vi "Plugin_GUI.vi"(8 "error in (no error)":errorcluster, 10 "Communication Interface":refnum<class "Communication Interface.lvclass">, 11 "Process in":refnum<class "Process.lvclass">) -> (0 "error out":errorcluster, 3 "Process out":refnum<class "Process.lvclass">)   [LabVIEW 2020, in "Plugin.lvlib" / "Plugin_UI.lvclass"]
doc: "Configuration User Interface for Plugin"
uses:
  Plugin_UI.lvclass
  builds/Libraries/Shared GUI Library.lvlibp/Shared GUI Library/Instrument Settings/Interface/Serial Interafce.ctl
  builds/Libraries/LabSys Framework.lvlibp/Process/Process/Process.lvclass
  builds/Libraries/LabSys Framework.lvlibp/Process/Communication Interface/Communication Interface.lvclass
  builds/Libraries/design.lvlibp/GUI/Design/CustomButtons/scale_32.ctl
  Output Channel Config.ctl
  builds/Libraries/Shared GUI Library.lvlibp/Shared GUI Library/Instrument Settings/Interface/Settings Container.ctl
  builds/Libraries/Shared GUI Library.lvlibp/Shared GUI Library/Device Meta Data Cluster/DeviceMetaDataCluster.ctl
  builds/Libraries/design.lvlibp/GUI/Design/CustomButtons/LineType/clear_list_l.ctl
  builds/Libraries/design.lvlibp/GUI/Design/CustomButtons/LineType/play_32.ctl
  builds/Libraries/Shared GUI Library.lvlibp/Shared GUI Library/Queue Driver/Typedefs/Operation.ctl
  builds/Libraries/LabSys Framework.lvlibp/Configurable Data Node/Configuration UI Event Interface/Configuration UI Event Interface.lvclass
  Main Cluster.ctl
  C:/SVN_LabSys/labsys_lvcode/LabSys_SourceCode/builds/Libraries/LabSys Framework.lvlibp/Configurable Data Node/Configuration Interface/Configuration Interface.lvclass
  C:/SVN_LabSys/labsys_lvcode/LabSys_SourceCode/builds/Libraries/LabSys Framework.lvlibp/Process/Process/Process.lvclass
  builds/Libraries/Shared GUI Library.lvlibp/Shared GUI Library/Producer error/Error type.ctl
  builds/Libraries/Shared GUI Library.lvlibp/1abvi3w/vi.lib/event_ctls.llb/lveventtype.ctl
  <vilib>/Utility/miscctls.llb/LVPointTypeDef.ctl
  builds/Libraries/LabSys Framework.lvlibp/Error Manager/Error Manager/Error Levels.ctl
  builds/Libraries/Shared GUI Library.lvlibp/Shared GUI Library/Queue Driver/Typedefs/Data.ctl
  Plugin_UI.lvclass/Plugin_UI.ctl
  builds/Libraries/Shared GUI Library.lvlibp/Shared GUI Library/Instrument Settings/Interface/Interface Type.ctl
  <vilib>/Utility/miscctls.llb/LVRowAndColumnTypeDef.ctl
  Write Input Channels[].vi
  Write Output Channels[].vi
  Read Output Channels[].vi
  Read Input Channels[].vi
  Channels/Output Channels/Output Channels.lvclass
  C:/SVN_LabSys/labsys_lvcode/LabSys_SourceCode/Plugin Template/Source/Code/Channels/Plugin_Channels.lvclass
  Channels/Input Channels/Input Channels.lvclass
  builds/Libraries/LabSys Framework.lvlibp/Configurable Data Node/Configuration Interface/Read Module Configuration.vi
  builds/Libraries/LabSys Framework.lvlibp/Configuration Storage/Module Configuration/Read Module Name.vi
  builds/Libraries/LabSys Framework.lvlibp/Configuration Storage/Module Configuration/Get Lookup Tables.vi
  builds/Libraries/LabSys Framework.lvlibp/Configuration Storage/Module Configuration/Get Scaling Functions.vi
  builds/Libraries/LabSys Framework.lvlibp/Configurable Data Node/Configuration Interface/Write Module Configuration.vi
  Write Lookup Tables.vi
  Write Scaling Functions.vi
  Read Lookup Tables.vi
  Read Scaling Functions.vi
  builds/Libraries/LabSys Framework.lvlibp/Configuration Storage/Module Configuration/Set Lookup Tables.vi
  builds/Libraries/LabSys Framework.lvlibp/Configuration Storage/Module Configuration/Set Scaling Functions.vi
  builds/Libraries/LabSys Framework.lvlibp/Process/Process/Read Error Manager.vi
  builds/Libraries/LabSys Framework.lvlibp/Configuration Storage/Module Configuration/Module Configuration.lvclass
  <vilib>/ErrorRing/Error Ring.xnode
  builds/Libraries/LabSys Framework.lvlibp/Error Manager/Error Manager/Error Manager.lvclass
  Controller_Class/Plugin_Controller.lvclass
  builds/Libraries/Shared GUI Library.lvlibp/Shared GUI Library/Queue Driver/Queue Driver.lvlib
  builds/Libraries/Shared GUI Library.lvlibp
  builds/Libraries/LabSys Framework.lvlibp/Configurable Data Node/Configuration Interface/Configuration Interface.lvclass
  C:/SVN_LabSys/labsys_lvcode/LabSys_SourceCode/builds/Libraries/LabSys Framework.lvlibp/Process/Communication Interface/Communication Interface.lvclass
  builds/Libraries/design.lvlibp
panel:
  in  "Label":string="Plugin_UI"
  in  "scale":T1
  in  "setDefault":bool
  in  "Tab Control":enum32{"Interface", "Channels", "Test"}(tab)
  in  "Timeout (ms)":i32=5000
  in  "VISA":refnum<visa-resource-name>
  in  "Device IP":string="192.168.1.1.100"
  in  "Device Meta Data":T2
  in  "Interface Type":T4=enum."Serial"
  in  "Serial Interface":T5={"Baud Rate"=9600, "Data Bits "=8, "Parity"=enum."None", "Stop Bits"=10} {"Stop Bits" items=["1.0", "1.5", "2.0"]; "Baud Rate" items=["1200"=1200, "2400"=2400, "4800"=4800, "9600"=9600, "19200"=19200, "38400"=38400, "57600"=57600, "115200"=115200]}
  in  "Refresh Time (ms)":dbl=1000.0 min=100.0 max=10000.0 step=10.0
  in  "Select All?":enum8{"False", "True", "Mixed"}(c332)
  in  "Measurement Channels":i32(listbox)=5
  in  "Output Settings":T6={"Enable Output"=FALSE, "Channel Name"="", "Value"=1.0, "Unit"=""} {"Value" min=-422.2 max=422.2 step=1.0 format="%#.1f"}
  in  "Start Test":T7 caption="Test"
  out "Test Result":i32(listbox)=-1
  # "#PluginSpecificEdits_UI_1 \nUpdate Plugin name"
  # "Hardware Configuration"
  # "#In Hardware Configuration controls are not locked Because #PluginSpecificEdits__UI_3"
  # "#PluginSpecificEdits_UI_2 \n1. Delete Hardware configuration Which is not required and update according to the \nInterface type"
  # "Device Meta Data"
  # "Input Settings"
  # "#PluginSpecificEdits_UI_16\n Add or Remove Pluginspecific parameters in O/P Settings"
  # "Output Settings"
  # "#PluginSpecificEdits_UI_24 \nHeader section based on available pluginSpecific Settings"
  # "Functional Test"
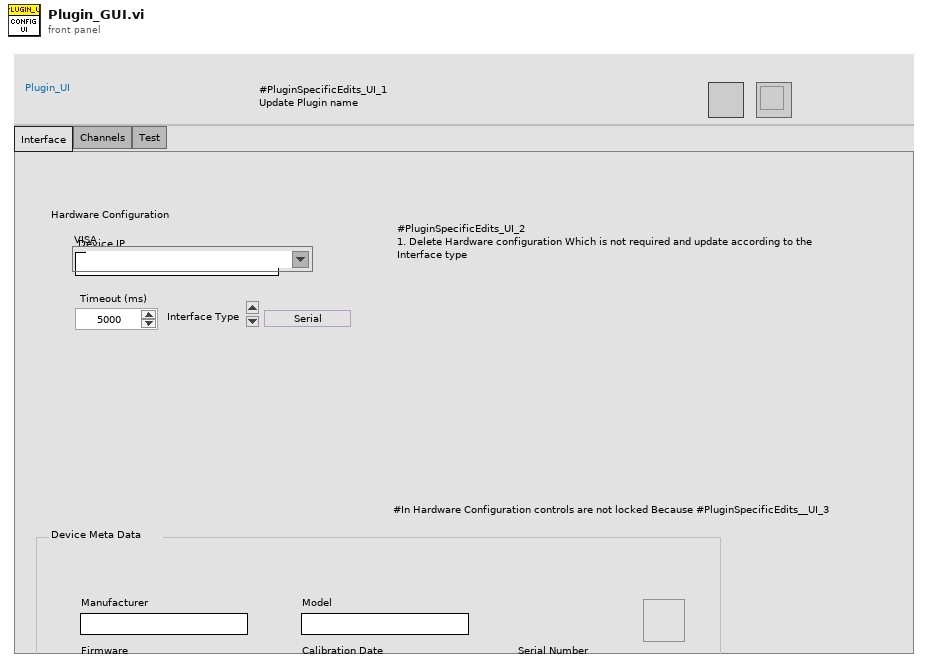
[diagram p1: front panel]
types:
  T1 = typedef "design.lvlibp/scale_32.ctl" = bool
  T2 = typedef "Shared GUI Library.lvlibp/DeviceMetaDataCluster.ctl" = cluster{"Manufacturer":string, "Model":string, "Serial Number":string, "Firmware":string, "Calibration Date":string, "Refresh":T3}
  T3 = typedef "design.lvlibp/clear_list_l.ctl" = bool
  T4 = typedef "Shared GUI Library.lvlibp/Settings Container.ctl" = enum32{"GPIB", "VXI", "GPIB-VXI", "Serial", "PXI", "TCPIP", "USB", "FireWire", "Invalid"}
  T5 = typedef "Shared GUI Library.lvlibp/Serial Interafce.ctl" = cluster{"Baud Rate":u32, "Data Bits ":u16, "Parity":enum16{"None", "Odd", "Even"}, "Stop Bits":u16}
  T6 = typedef "Plugin.lvlib/Plugin_UI.lvclass/Output Channel Config.ctl" = cluster{"Enable Output":bool, "Channel Name":string, "Value":dbl, "Unit":string}
  T7 = typedef "design.lvlibp/play_32.ctl" = bool
  T8 = typedef "LVPointTypeDef.ctl" = cluster{"Horizontal":i16, "Vertical":i16}
  T9 = typedef "Shared GUI Library.lvlibp/Error type.ctl" = cluster{"Type":T10, "Ctl Refnum":refnum<vi>}
  T10 = typedef "Shared GUI Library.lvlibp/lveventtype.ctl" = enum32{"Null", "Timeout", "Annotation Menu Selection", "Annotation Menu Selection?", "App Instance Close", "App Instance Close?", "Autoscale Range Change", "Bookmark Info Change", "Cell Edit", "Cell Edit?", "Cursor Grab", "Cursor Grab?", "Cursor Menu Selection", "Cursor Menu Selection?", "Cursor Move", "Cursor Release", "Data Change", "Direction Change", "Display State Change", "Drag Ended", "Drag Enter", "Drag Leave", "Drag Over", "Drag Source Update", "Drag Starting", "Drag Starting?", "Drop", "Exec State Change", "Key Down", "Key Down?", "Key Repeat", "Key Repeat?", "Key Up", "Listbox Double Click", "Menu Activation?", "Menu Selection (App)", "Menu Selection? (App)", "Menu Selection (User)", "Mouse Down", "Mouse Down?", "Mouse Enter", "Mouse Leave", "Mouse Move", "Mouse Up", "Mouse Wheel", "NI Security User Change (App)", "Pane Size", "Panel Close", "Panel Close?", "Panel Resize", "Plot Attribute Change", "Scale Range Change", "Shortcut Menu Activation?", "Shortcut Menu Selection (App)", "Shortcut Menu Selection? (App)", "Shortcut Menu Selection (User)", "Tree Double Click", "Tree Drag", "Tree Drag?", "Tree Drop", "Tree Drop?", "Tree Item Close", "Tree Item Close?", "Tree Item Open", "Tree Item Open?", "User Event", "Value Change"}
  T11 = typedef "Plugin.lvlib/Plugin_UI.lvclass/Main Cluster.ctl" = cluster{"Current Config":refnum<class "Plugin_UI.lvclass">, "Initial Config":refnum<class "Plugin_UI.lvclass">, "Change Flag":bool, "Output Ch. Name":string, "Input Ch. Name[]":string[], "No. of Input Ch.":i32, "Default Ch. Status":bool, "Output Status":bool, "Plugin Name":string}
  T12 = typedef "Shared GUI Library.lvlibp/Queue Driver.lvlib/Operation.ctl" = enum16{"Create", "Enqueue without Data", "Enstack without Data", "Enqueue N Elements without Data", "Enqueue with Data", "Enstack with Data", "Enqueue N Elements with Data", "Dequeue", "Flush", "Release"}
  T13 = typedef "Shared GUI Library.lvlibp/Queue Driver.lvlib/Data.ctl" = cluster{"State":string, "Data":variant}
  T14 = typedef "lveventtype.ctl" = enum32{"Null", "Timeout", "Annotation Menu Selection", "Annotation Menu Selection?", "App Instance Close", "App Instance Close?", "Autoscale Range Change", "Bookmark Info Change", "Cell Edit", "Cell Edit?", "Cursor Grab", "Cursor Grab?", "Cursor Menu Selection", "Cursor Menu Selection?", "Cursor Move", "Cursor Release", "Data Change", "Direction Change", "Display State Change", "Drag Ended", "Drag Enter", "Drag Leave", "Drag Over", "Drag Source Update", "Drag Starting", "Drag Starting?", "Drop", "Exec State Change", "Key Down", "Key Down?", "Key Repeat", "Key Repeat?", "Key Up", "Listbox Double Click", "Menu Activation?", "Menu Selection (App)", "Menu Selection? (App)", "Menu Selection (User)", "Mouse Down", "Mouse Down?", "Mouse Enter", "Mouse Leave", "Mouse Move", "Mouse Up", "Mouse Wheel", "NI Security User Change (App)", "Pane Size", "Panel Close", "Panel Close?", "Panel Resize", "Plot Attribute Change", "Scale Range Change", "Shortcut Menu Activation?", "Shortcut Menu Selection (App)", "Shortcut Menu Selection? (App)", "Shortcut Menu Selection (User)", "Tree Double Click", "Tree Drag", "Tree Drag?", "Tree Drop", "Tree Drop?", "Tree Item Close", "Tree Item Close?", "Tree Item Open", "Tree Item Open?", "User Event", "Value Change"}
  T15 = typedef "LabSys Framework.lvlibp/Configurable Data Node.lvlib/Configuration Interface.lvclass/UI Events.ctl" = enum8{"Stop", "Save Content", "Invoke Plugin", "Custom Message", "Update Initial Config", "ScalingEnabled?", "ScalingDisabled"}
  T16 = typedef "LVRowAndColumnTypeDef.ctl" = cluster{"Row":i32, "Column":i32}
  T17 = typedef "LVPoint32TypeDef.ctl" = cluster{"Horizontal":i32, "Vertical":i32}
  T18 = typedef "LabSys Framework.lvlibp/Error Manager.lvlib/Error Manager.lvclass/Error Levels.ctl" = enum8{"Warning", "Error", "Fatal Error"}
  T19 = enum8{"Enabled", "Disabled", "Disabled and Grayed Out"}
  T20 = typedef "LabSys Framework.lvlibp/Configuration Storage.lvlib/Test Configuration.lvclass/Table Information.ctl" = cluster{"Name":string, "Lookup Table":dbl[][]}
  T21 = typedef "LabSys Framework.lvlibp/Configuration Storage.lvlib/Test Configuration.lvclass/Function Information.ctl" = cluster{"Name":string, "Expression":string, "Constants":T22[], "Test Data":dbl[][]}
  T22 = typedef "LabSys Framework.lvlibp/Configuration Storage.lvlib/Test Configuration.lvclass/Function Constant Value.ctl" = cluster{"Constant Name":string, "Value":dbl}
  T23 = typedef "Plugin.lvlib/Plugin_UI.lvclass/UDP Configuration.ctl" = cluster{"Device Port Number":u16, "Device IP":string, "Timeout":i32, "Port Number":u16}
  T24 = typedef "Plugin.lvlib/Plugin_UI.lvclass/Serial Configuration.ctl" = cluster{"VISA":refnum<visa-resource-name>, "Interface Type":T25, "Serial Interface":T5, "Slave Address":u8}
  T25 = typedef "Shared GUI Library.lvlibp/Interface Type.ctl" = u16
  T26 = typedef "LabSys Framework.lvlibp/Configuration Storage.lvlib/Test Configuration.lvclass/Scaling Information.ctl" = cluster{"Active":bool, "Scaling Type":T27, "Output Minimum":dbl, "Output Maximum":dbl, "Raw Minimum":dbl, "Raw Maximum":dbl, "Output Unit":string, "Function":string, "Lookup Table":string}
  T27 = typedef "LabSys Framework.lvlibp/Configuration Storage.lvlib/Test Configuration.lvclass/Scaling Types.ctl" = enum8{"Linear", "Function", "Lookup Table"}
  T28 = typedef "LabSys Framework.lvlibp/Data Node.lvlib/Data Node.lvclass/Result.ctl" = cluster{"Result Type":T29, "Explanation":string}
  T29 = typedef "LabSys Framework.lvlibp/Data Node.lvlib/Data Node.lvclass/Result Type.ctl" = enum16{"Information", "Warning", "Error"}
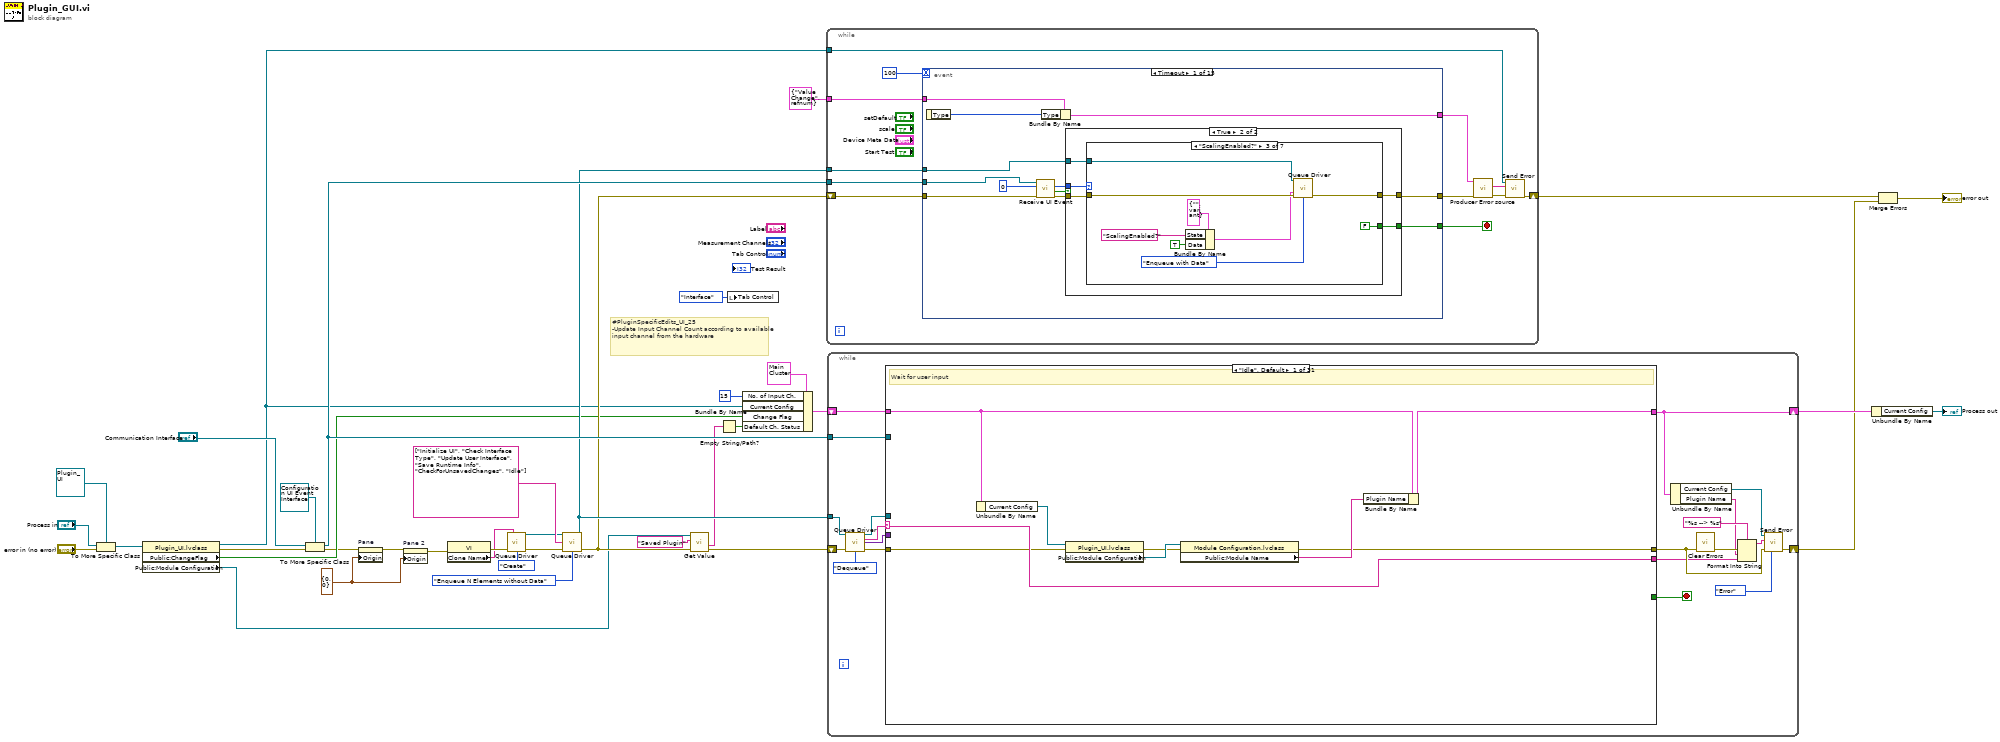
[diagram p0: block diagram]
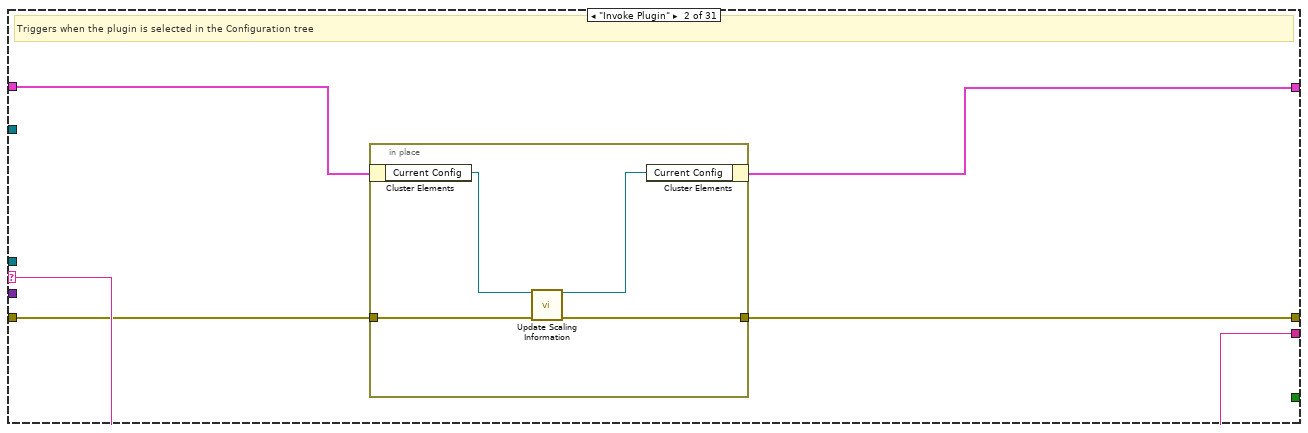
[diagram p2: hidden frame]
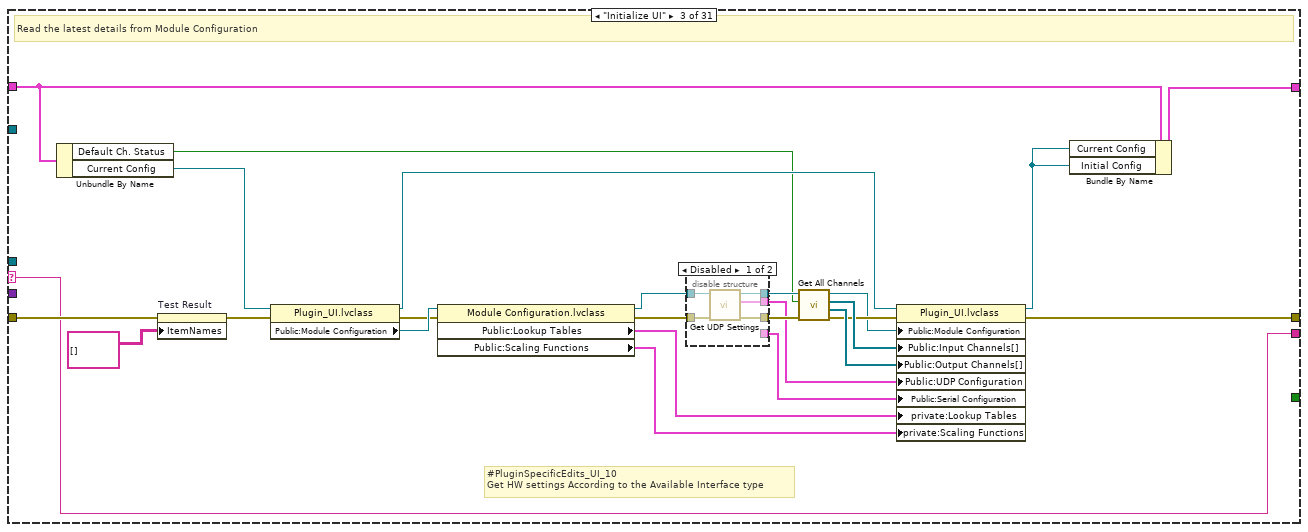
[diagram p3: hidden frame]
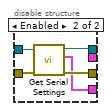
[diagram p4: hidden frame]
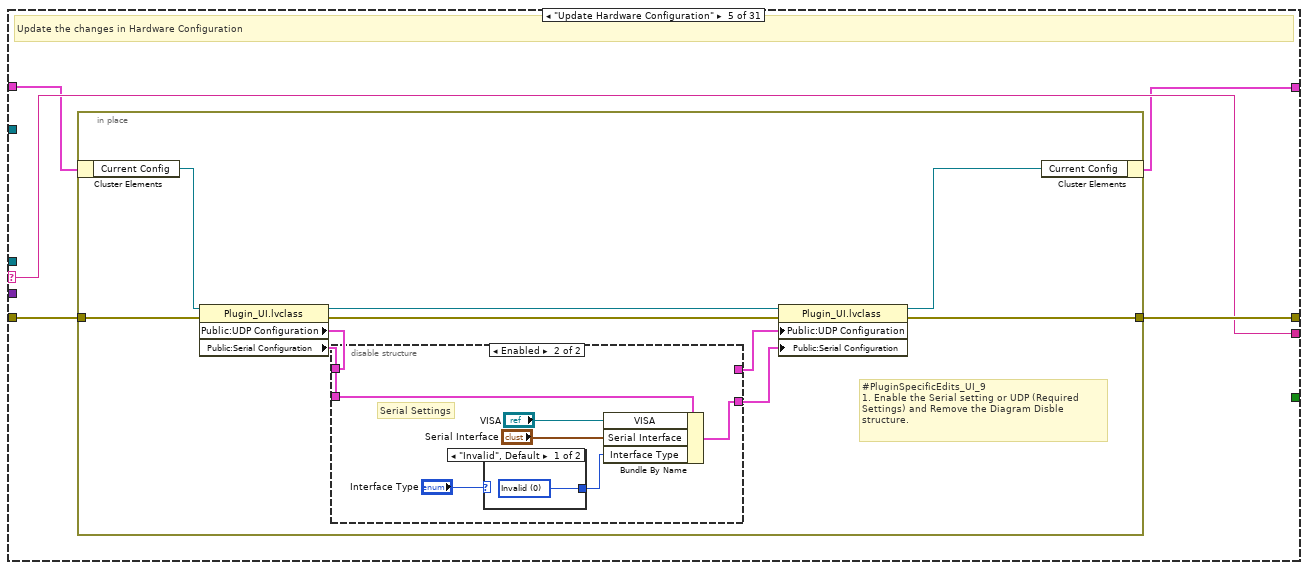
[diagram p6: hidden frame]
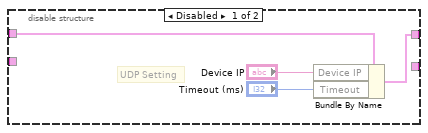
[diagram p7: hidden frame]
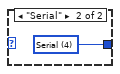
[diagram p8: hidden frame]
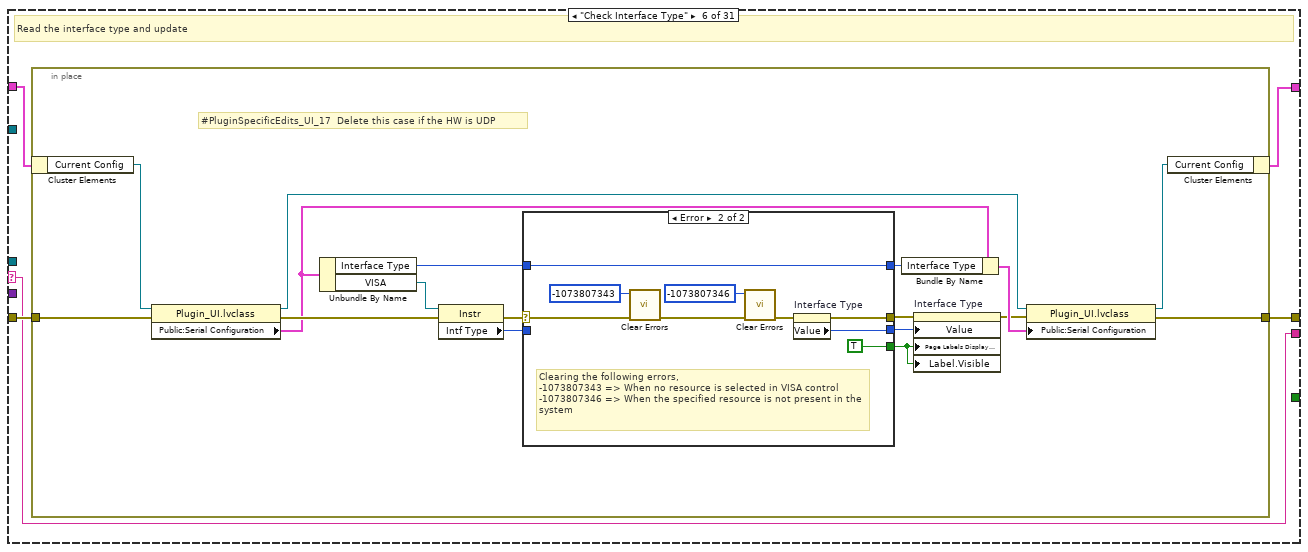
[diagram p9: hidden frame]
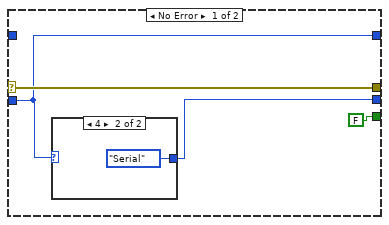
[diagram p10: hidden frame]
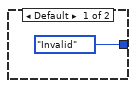
[diagram p11: hidden frame]
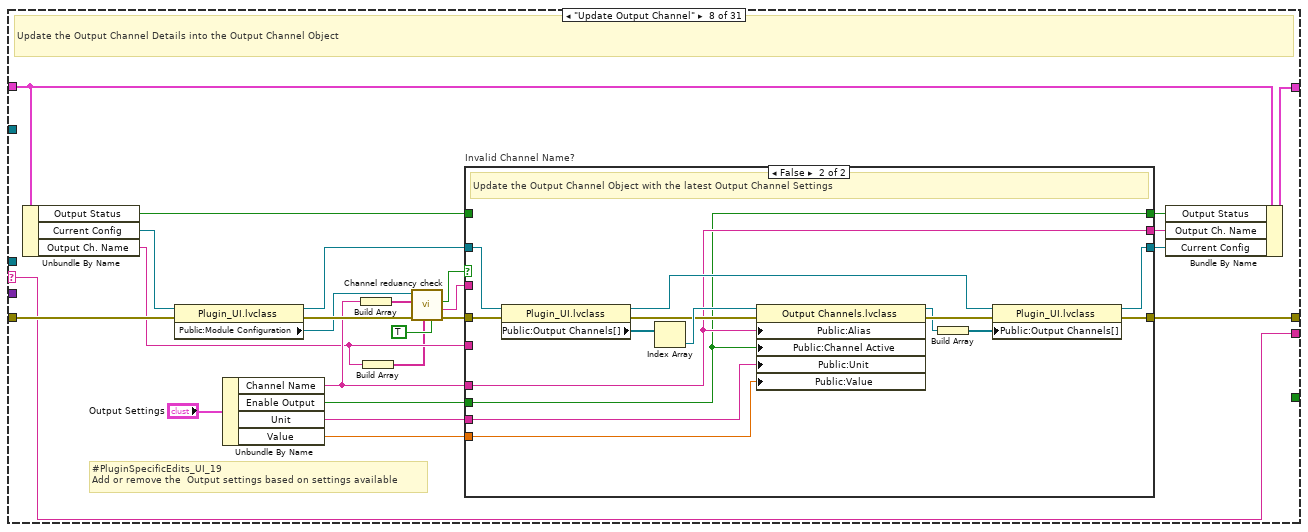
[diagram p13: hidden frame]
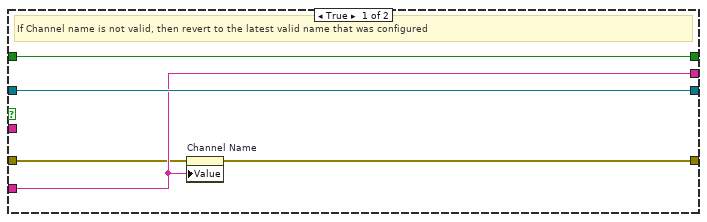
[diagram p14: hidden frame]
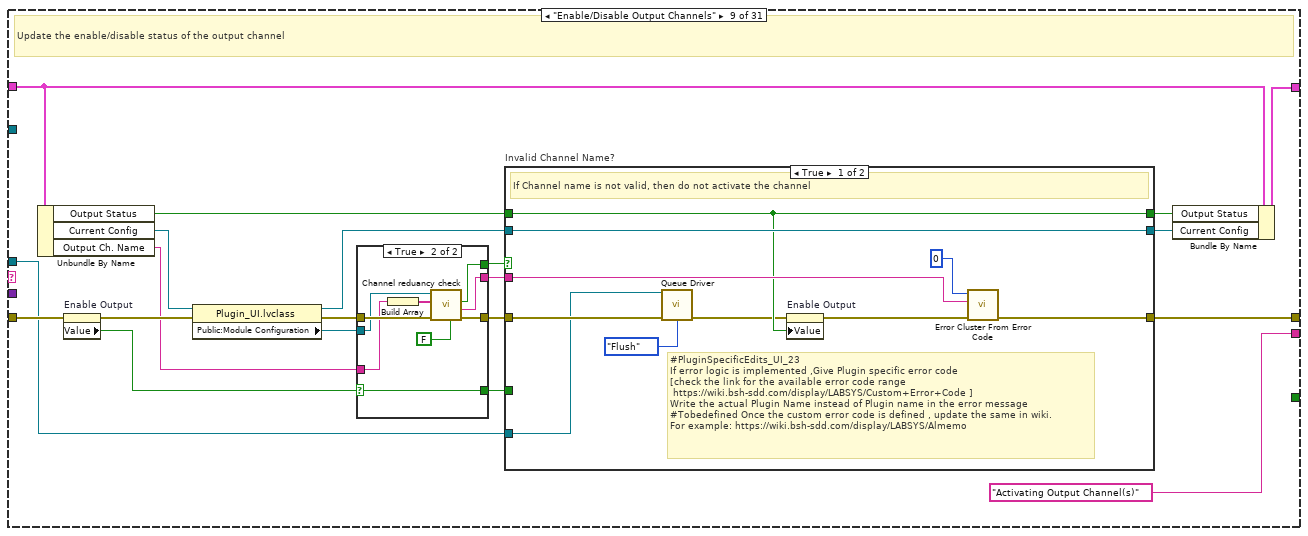
[diagram p15: hidden frame]
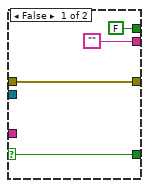
[diagram p16: hidden frame]
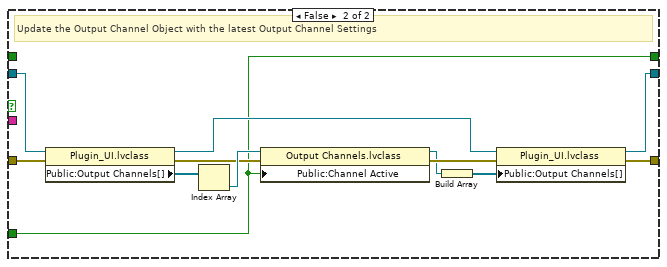
[diagram p17: hidden frame]
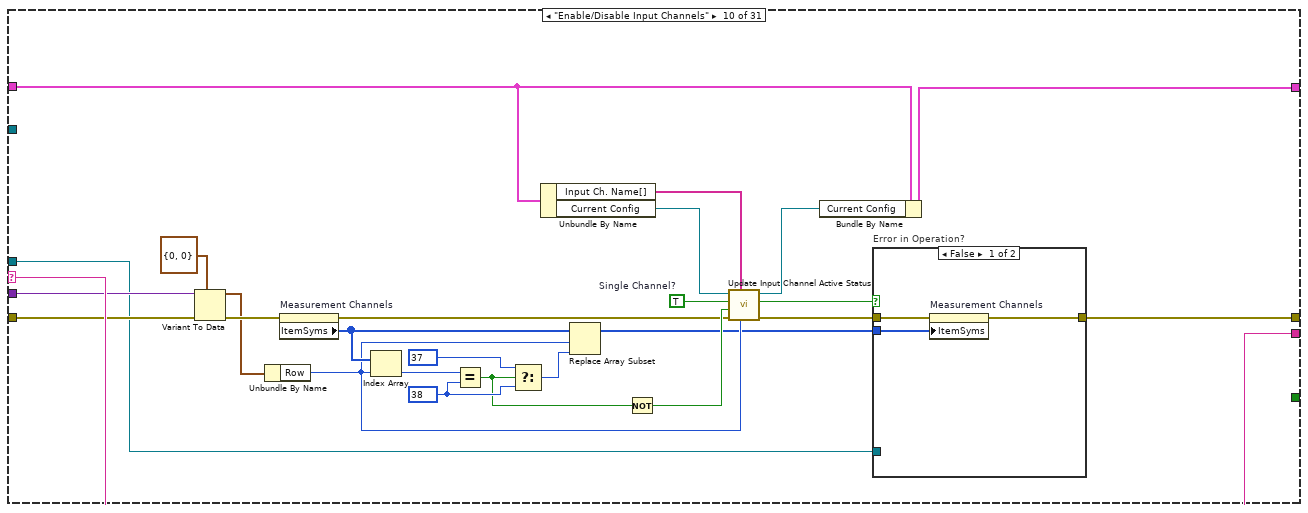
[diagram p18: hidden frame]
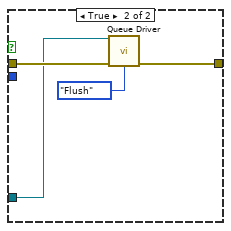
[diagram p19: hidden frame]
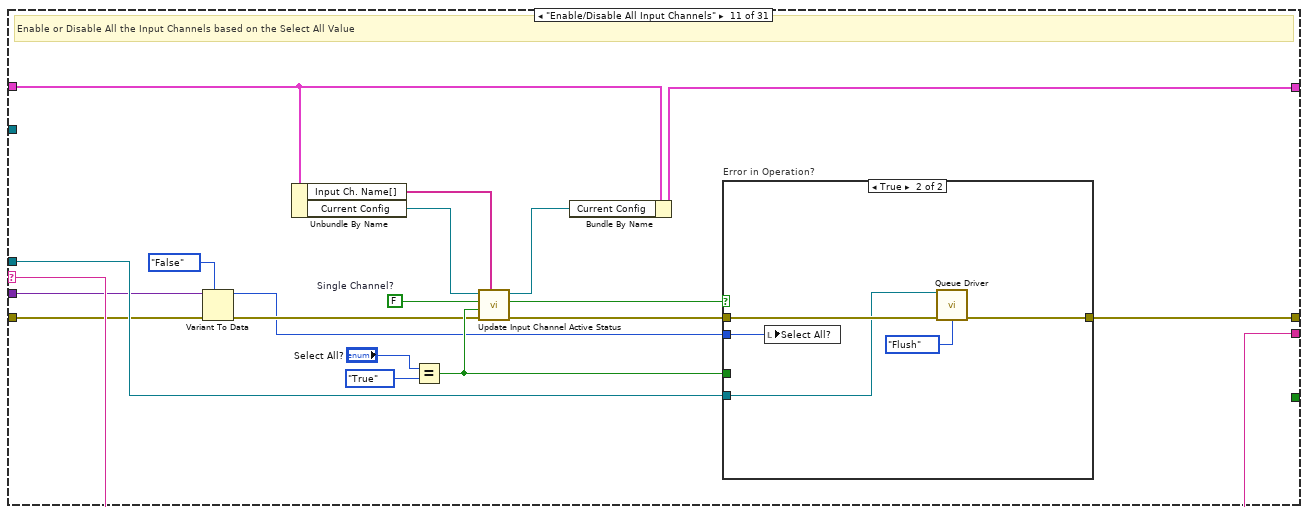
[diagram p20: hidden frame]
diagram:
  w4 = T8 {"Horizontal"=0, "Vertical"=0} ("Origin")
  # "#PluginSpecificEdits_UI_25\n-Update Input Channel Count according to available input channel from the hardware"
  n1 = To More Specific Class(target class=refnum<class "Plugin_UI.lvclass"> refnum ("Plugin.lvlib:Plugin_UI.lvclass"), reference="Process in", error in="error in (no error)") -> (specific class reference=w5:refnum<class "Plugin_UI.lvclass">)  [unwired: 1 out]
  n2 = property on="Property Node" class="Plugin_UI.lvclass"(reference=w5) -> (reference out=w19:refnum<class "Plugin_UI.lvclass">, error out=w21:errorcluster, "Public:ChangeFlag"=w7:bool, "Public:Module Configuration"=w12:refnum<class "Module Configuration.lvclass">)  [unwired: 1 in]
  n3 = To More Specific Class(target class=refnum<class "Configuration UI Event Interface.lvclass"> refnum ("LabSys Framework.lvlibp:Configurable Data Node.lvlib:Configuration UI Event Interface.lvclass"), reference="Communication Interface", error in=w21) -> (specific class reference=w36:refnum<class "Configuration UI Event Interface.lvclass">, error out=w1:errorcluster)
  n4 = property on="Pane" class="Pane"(error in=w1, "Origin"=w4) -> (error out=w6:errorcluster)  [unwired: 1 in, 1 out]
  n5 = property on="Pane 2" class="Pane"(error in=w6, "Origin"=w4) -> (error out=w2:errorcluster)  [unwired: 1 in, 1 out]
  n6 = property on="Property Node" class="VI"(error in=w2) -> (error out=w33:errorcluster, "Clone Name"=w32:string)  [unwired: 1 in, 1 out]
  n7 = call "Queue Driver.vi"("Queue Name"=w32, "error in (no error)"=w33, "Operation"=Operation."Create") -> ("Queue Out"=w28:refnum<queue>, "error out"=w31:errorcluster)  [unwired: 9 in, 2 out]
  n8 = call "Queue Driver.vi"("Queue In"=w28, "State[]"=string[] ["Initialize UI", "Check Interface Type", "Update User Interface", "Save Runtime Info", "CheckForUnsavedChanges", "Idle"], "error in (no error)"=w31, "Operation"=Operation."Enqueue N Elements without Data") -> ("Queue Out"=w26:refnum<queue>, "error out"=w20:errorcluster)  [unwired: 8 in, 2 out]
  n9 = call "Get Value.vi"("error in (no error)"=w20, "Key"="Saved Plugin", "Module Configuration in"=w12) -> ("error out"=w3:errorcluster, "Value"=w10:string)  [unwired: 6 in, 1 out]
  n10 = Empty String/Path?(string/path=w10) -> (empty?=w9:bool)
  n11 = local write "Tab Control"(enum32{"Interface", "Channels", "Test"}."Interface" ("Tab Control")) -> ()
  n12 = Bundle By Name(cluster=T11 {"Current Config"=refnum, "Initial Config"=refnum, "Change Flag"=FALSE, "Output Ch. Name"="", "Input Ch. Name[]"=[], "No. of Input Ch."=0, "Default Ch. Status"=FALSE, "Output Status"=FALSE, "Plugin Name"=""}, "No. of Input Ch."=15, "Current Config"=w19, "Change Flag"=w7, "Default Ch. Status"=w9) -> (w24:T11)
  n13 = while {
    shift-right: [w43] -> w16
    shift-left: w20 -> [w49]
    tunnel: w36 -> [w48]
    tunnel: w26 -> [w47]
    tunnel: w19 -> [w40]
    tunnel: T9 {"Type"=enum."Value Change", "Ctl Refnum"=refnum} ("Cluster") -> [w39]
    stop <- w46 stop-if-true
    n14 = event shown="[0] Timeout" {
      selector: _ -> [_ _ _ _ _ _ _ _ _ _ _ _ _ _ _]
      dyn-events: _ -> [_ _ _ _ _ _ _ _ _ _ _ _ _ _ _]
      timeout: 100 -> [_ _ _ _ _ _ _ _ _ _ _ _ _ _ _]
      tunnel: [w61 _ _ _ _ _ _ _ _ _ _ _ _ _ _] -> w46
      tunnel: [w62 w120 w129 w136 w145 w156 w160 w174 w183 w192 w212 w217 w227 w268 w277] -> w45
      tunnel: w49 -> [w58 w121 w130 w138 w147 w157 w161 w175 w184 w193 w202 w219 w230 w269 w279]
      tunnel: w48 -> [w60 _ _ _ _ _ _ _ _ _ _ _ _ _ _]
      tunnel: w47 -> [w54 w119 w128 w137 w146 w155 w162 w173 w182 w191 w211 w214 w222 w270 w278]
      tunnel: w39 -> [w53 w118 w127 w133 w143 w154 w167 w172 w181 w190 w210 w221 w234 w267 w276]
      tunnel: [w51 w115 w124 w132 w142 w151 w164 w170 w179 w188 w208 w218 w233 w264 w273] -> w42
      event Timeout {
        n15 = event-data() -> ("Type"=w52:T14)  [unwired: 1 in]
        n16 = call "Receive UI Event.vi"("error in (no error)"=w58, "Timeout"=0, "Communication Interface in"=w60) -> ("error out"=w56:errorcluster, "Event Valid"=w59:bool, "UI Event"=w55:T15)  [unwired: 5 in, 1 out]
        n17 = Bundle By Name(cluster=w53, "Type"=w52) -> (w51:T9)
        n18 = case shown="True" w59 {
          tunnel: [w63 w67] -> w62
          tunnel: [FALSE w66] -> w61
          tunnel: w56 -> [w63 w65]
          tunnel: w55 -> [_ w69]
          tunnel: w54 -> [_ w68]
          frame False {
          }
          frame True {
            n19 = case shown="\"ScalingEnabled?\"" w69 {
              tunnel: w65 -> [w71 w81 w90 w95 w101 w104 w110]
              tunnel: [w73 w83 w92 w94 w101 w103 w109] -> w67
              tunnel: w68 -> [w72 w82 w91 w96 _ w105 w111]
              tunnel: [FALSE FALSE FALSE TRUE FALSE FALSE FALSE] -> w66
              frame "Save Content" {
                n20 = call "Queue Driver.vi"("Queue In"=w72, "State[]"=string[] ["Save Runtime Info", "Send Save Response"], "error in (no error)"=w71, "Operation"=Operation."Enqueue N Elements without Data") -> ("error out"=w73:errorcluster)  [unwired: 8 in, 3 out]
              }
              frame "ScalingDisabled" {
                n21 = Bundle By Name(cluster=T13 {"State"="", "Data"=variant} ("State with Data"), "State"="ScalingEnabled?", "Data"=FALSE) -> (w76:T13)
                n22 = call "Queue Driver.vi"("Queue In"=w82, "State with Data"=w76, "error in (no error)"=w81, "Operation"=Operation."Enqueue with Data") -> ("error out"=w83:errorcluster)  [unwired: 8 in, 3 out]
              }
              frame "ScalingEnabled?" {
                n23 = Bundle By Name(cluster=T13 {"State"="", "Data"=variant} ("State with Data"), "State"="ScalingEnabled?", "Data"=TRUE) -> (w85:T13)
                n24 = call "Queue Driver.vi"("Queue In"=w91, "State with Data"=w85, "error in (no error)"=w90, "Operation"=Operation."Enqueue with Data") -> ("error out"=w92:errorcluster)  [unwired: 8 in, 3 out]
              }
              frame "Stop" {
                n25 = call "Queue Driver.vi"("Queue In"=w96, "State"="Stop", "error in (no error)"=w95, "Operation"=Operation."Enqueue without Data") -> ("error out"=w94:errorcluster)  [unwired: 8 in, 3 out]
              }
              frame "Custom Message" {
              }
              frame "Invoke Plugin" {
                n26 = call "Queue Driver.vi"("Queue In"=w105, "State[]"=string[] ["Invoke Plugin", "CheckForUnsavedChanges", "Update User Interface"], "error in (no error)"=w104, "Operation"=Operation."Enqueue N Elements without Data") -> ("error out"=w103:errorcluster)  [unwired: 8 in, 3 out]
              }
              frame "Update Initial Config" {
                n27 = call "Queue Driver.vi"("Queue In"=w111, "State[]"=string[] ["Update Initial Config", "Send Save Response"], "error in (no error)"=w110, "Operation"=Operation."Enqueue N Elements without Data") -> ("error out"=w109:errorcluster)  [unwired: 8 in, 3 out]
              }
            }
          }
        }
      }
      event Value Change {
        n28 = event-data() -> ("Type"=w117:T14, "CtlRef"=w116:refnum<vi>)  [unwired: 1 in]
        n29 = Bundle By Name(cluster=w118, "Type"=w117, "Ctl Refnum"=w116) -> (w115:T9)
        n30 = call "Queue Driver.vi"("Queue In"=w119, "State[]"=string[] ["Consistency Check", "Test"], "error in (no error)"=w121, "Operation"=Operation."Enqueue N Elements without Data") -> ("error out"=w120:errorcluster)  [unwired: 8 in, 3 out]
      }
      event "Device IP", "Timeout (ms)": Value Change {
        # "#PluginSpecificEdits_UI_4\nDelete the UDP Setting and follow the steps,  If not required UDP Hardware settings\n1. Goto \"Update Hardware Configuration\" case, and Enable the Serial settings and Remove the Diagram Disble structure.\n2. Goto \"Save Runtime Info\" Case, Enable the \"SET SERIAL SETTING vi\" and Remove the Diagram Disble structure. \n3. Goto \"CheckForUnsavedChanges\" case,  Open Check for Unsaved chnages Changes Vi\n3.1 Delete the Comparision for the UDP Settings\n4. Delete the UDP Event case. 5. Delete respected Hardware settings from Private class and Update in the Cases"
        n31 = event-data() -> ("Type"=w126:T14, "CtlRef"=w125:refnum<vi>)  [unwired: 1 in]
        n32 = Bundle By Name(cluster=w127, "Type"=w126, "Ctl Refnum"=w125) -> (w124:T9)
        n33 = call "Queue Driver.vi"("Queue In"=w128, "State[]"=string[] ["Update Hardware Configuration", "Save Runtime Info", "CheckForUnsavedChanges"], "error in (no error)"=w130, "Operation"=Operation."Enqueue N Elements without Data") -> ("error out"=w129:errorcluster)  [unwired: 8 in, 3 out]
      }
      event Value Change {
        # "#PluginSpecificEdits_UI_5 \nDelete theSerial Setting and follow the steps,  If not required Serial Hardware settings\n1. Goto \"Update Hardware Configuration\" case, and Enable the UDP settings and Remove the Diagram Disble structure.\n2. Goto  \"Save Runtime Info\", Enable the \"SET UDP SETTING vi\" and Remove the Diagram Disble structure.\n3. Goto \"CheckForUnsavedChanges\" case,  Open Check for Unsaved chnages Changes Vi\n3.1 Delete the Comparision for theSerial Settings\n4. Delete Setial Setting Event case. 5. Delete respected Hardware settings from Private class and Update in the Cases"
        n34 = event-data() -> ("Type"=w135:T14, "CtlRef"=w134:refnum<vi>)  [unwired: 1 in]
        n35 = Bundle By Name(cluster=w133, "Type"=w135, "Ctl Refnum"=w134) -> (w132:T9)
        n36 = call "Queue Driver.vi"("Queue In"=w137, "State[]"=string[] ["Update Hardware Configuration", "Save Runtime Info", "CheckForUnsavedChanges"], "error in (no error)"=w138, "Operation"=Operation."Enqueue N Elements without Data") -> ("error out"=w136:errorcluster)  [unwired: 8 in, 3 out]
      }
      event "VISA": Value Change {
        # "#PluginSpecificEdits_UI_17  Delete this case if the HW is UDP"
        n37 = event-data() -> ("Type"=w144:T14, "CtlRef"=w141:refnum<vi>)  [unwired: 1 in]
        n38 = Bundle By Name(cluster=w143, "Type"=w144, "Ctl Refnum"=w141) -> (w142:T9)
        n39 = call "Queue Driver.vi"("Queue In"=w146, "State[]"=string[] ["Update Hardware Configuration", "Check Interface Type", "Save Runtime Info", "CheckForUnsavedChanges"], "error in (no error)"=w147, "Operation"=Operation."Enqueue N Elements without Data") -> ("error out"=w145:errorcluster)  [unwired: 8 in, 3 out]
      }
      event "Refresh Time (ms)": Value Change {
        n40 = event-data() -> ("Type"=w153:T14, "CtlRef"=w152:refnum<vi>)  [unwired: 1 in]
        n41 = Bundle By Name(cluster=w154, "Type"=w153, "Ctl Refnum"=w152) -> (w151:T9)
        n42 = call "Queue Driver.vi"("Queue In"=w155, "State[]"=string[] ["Update Refresh Time", "Save Runtime Info", "CheckForUnsavedChanges"], "error in (no error)"=w157, "Operation"=Operation."Enqueue N Elements without Data") -> ("error out"=w156:errorcluster)  [unwired: 8 in, 3 out]
      }
      event Value Change {
        n43 = event-data() -> ("Type"=w166:T14, "CtlRef"=w165:refnum<vi>)  [unwired: 1 in]
        n44 = Bundle By Name(cluster=w167, "Type"=w166, "Ctl Refnum"=w165) -> (w164:T9)
        n45 = call "Queue Driver.vi"("Queue In"=w162, "State[]"=string[] ["Get Device Meta Data", "Save Runtime Info", "CheckForUnsavedChanges"], "error in (no error)"=w161, "Operation"=Operation."Enqueue N Elements without Data") -> ("error out"=w160:errorcluster)  [unwired: 8 in, 3 out]
      }
      event Value Change {
        n46 = event-data() -> ("Type"=w171:T14, "CtlRef"=w169:refnum<vi>)  [unwired: 1 in]
        n47 = Bundle By Name(cluster=w172, "Type"=w171, "Ctl Refnum"=w169) -> (w170:T9)
        n48 = call "Queue Driver.vi"("Queue In"=w173, "State[]"=string[] ["Update Output Channel", "Save Runtime Info", "CheckForUnsavedChanges"], "error in (no error)"=w175, "Operation"=Operation."Enqueue N Elements without Data") -> ("error out"=w174:errorcluster)  [unwired: 8 in, 3 out]
      }
      event Value Change {
        n49 = event-data() -> ("Type"=w180:T14, "CtlRef"=w178:refnum<vi>)  [unwired: 1 in]
        n50 = Bundle By Name(cluster=w181, "Type"=w180, "Ctl Refnum"=w178) -> (w179:T9)
        n51 = call "Queue Driver.vi"("Queue In"=w182, "State[]"=string[] ["Update Output Channel", "Update User Interface", "Save Runtime Info", "CheckForUnsavedChanges"], "error in (no error)"=w184, "Operation"=Operation."Enqueue N Elements without Data") -> ("error out"=w183:errorcluster)  [unwired: 8 in, 3 out]
      }
      event Value Change {
        n52 = event-data() -> ("Type"=w189:T14, "CtlRef"=w187:refnum<vi>)  [unwired: 1 in]
        n53 = Bundle By Name(cluster=w190, "Type"=w189, "Ctl Refnum"=w187) -> (w188:T9)
        n54 = call "Queue Driver.vi"("Queue In"=w191, "State[]"=string[] ["Enable/Disable Output Channels", "Save Runtime Info", "CheckForUnsavedChanges"], "error in (no error)"=w193, "Operation"=Operation."Enqueue N Elements without Data") -> ("error out"=w192:errorcluster)  [unwired: 8 in, 3 out]
      }
      event "Select All?": Value Change {
        n55 = event-data() -> ("Type"=w209:T14, "CtlRef"=w207:refnum<vi>, "NewVal"=w204:enum8{"False", "True", "Mixed"}, "OldVal"=w200:enum8{"False", "True", "Mixed"})  [unwired: 1 in]
        n56 = Equal?(x=w204, y=enum8{"False", "True", "Mixed"}."True") -> (x = y?=w205:bool)
        n57 = Select(t=w204, s=w205, f=enum8{"False", "True", "Mixed"}."False" ("y")) -> (s? t:f=w195:enum8{"False", "True", "Mixed"})
        n58 = local write "Select All?"(w195) -> ()
        n59 = Bundle By Name(cluster=w210, "Type"=w209, "Ctl Refnum"=w207) -> (w208:T9)
        n60 = To Variant(anything=w200) -> (Variant=w198:variant)
        n61 = Bundle By Name(cluster=T13 {"State"="Enable/Disable All Input Channels", "Data"=variant} ("State with Data"), "Data"=w198) -> (w196:T13)
        n62 = Build Array (concatenate)(w196, T13[] [{"State"="Save Runtime Info", "Data"=variant}, {"State"="CheckForUnsavedChanges", "Data"=variant}] ("State with Data[]")) -> (w197:T13[])
        n63 = call "Queue Driver.vi"("Queue In"=w211, "error in (no error)"=w202, "State with Data[]"=w197, "Operation"=Operation."Enqueue N Elements with Data") -> ("error out"=w212:errorcluster)  [unwired: 8 in, 3 out]
      }
      event "Measurement Channels": Edit Cell {
        n64 = event-data() -> ("Type"=w220:T14, "CtlRef"=w216:refnum<vi>, "Coords"=w215:T16)  [unwired: 1 in]
        n65 = call "Identify Measurement Channel Edits.vi"("Queue Ref"=w214, "Coords"=w215, "error in (no error)"=w219) -> ("error out"=w217:errorcluster)  [unwired: 11 in, 1 out]
        n66 = Bundle By Name(cluster=w221, "Type"=w220, "Ctl Refnum"=w216) -> (w218:T9)
      }
      event "Measurement Channels": Mouse Up {
        n67 = event-data() -> ("Type"=w232:T14, "CtlRef"=w231:refnum<vi>, "Coords"=w228:T17)  [unwired: 1 in]
        n68 = invoke on="Invoke Node" class="MCListbox (strict)" method="Point To Row Column"(reference=w231, error in=w230, "Point"=w228) -> (reference out=w225:refnum<vi>, error out=w226:errorcluster, "CellPosition"=w224:T16, "InGlyph"=w223:bool)  [unwired: 4 in, 3 out]
        n69 = case "If the symbol cell is selected?" shown="False" w223 {
          tunnel: [w238 w263] -> w229
          tunnel: [w237 w262] -> w227
          tunnel: w226 -> [w240 w261]
          tunnel: w225 -> [w239 w263]
          tunnel: w224 -> [w235 w260]
          tunnel: w222 -> [_ w259]
          frame False {
            n70 = Unbundle By Name(w235) -> ("Row"=w236:i32, "Column"=w242:i32)
            n71 = In Range and Coerce(upper limit=2, x=w242, lower limit=1) -> (In Range?=w241:bool)  [unwired: 1 out]
            n72 = case "If the 1st or 2nd col is selected?" shown="False" w241 {
              tunnel: w240 -> [w245 w251]
              tunnel: w239 -> [w246 w252]
              tunnel: [w246 w250] -> w238
              tunnel: [w245 w249] -> w237
              tunnel: w236 -> [_ w248]
              tunnel: w235 -> [_ w247]
              frame False {
              }
              frame True {
                n73 = property on="Property Node" class="MCListbox (strict)"(reference=w252, error in=w251, "EditPos"=w247, "Value"=w248) -> (reference out=w250:refnum<vi>, error out=w249:errorcluster)
              }
            }
          }
          frame True {
            n74 = Bundle(cluster=T13 {"State"="", "Data"=variant} ("State with Data"), "State"="Enable/Disable Input Channels", "Data"=w260) -> (w255:T13)
            n75 = Build Array (concatenate)(w255, T13[] [{"State"="Save Runtime Info", "Data"=variant}, {"State"="CheckForUnsavedChanges", "Data"=variant}, {"State"="Update User Interface", "Data"=variant}] ("State with Data[]")) -> (w253:T13[])
            n76 = call "Queue Driver.vi"("Queue In"=w259, "error in (no error)"=w261, "State with Data[]"=w253, "Operation"=Operation."Enqueue N Elements with Data") -> ("error out"=w262:errorcluster)  [unwired: 8 in, 3 out]
          }
        }
        n77 = Bundle By Name(cluster=w234, "Type"=w232, "Ctl Refnum"=w229) -> (w233:T9)
      }
      event Value Change {
        n78 = event-data() -> ("Type"=w266:T14, "CtlRef"=w265:refnum<vi>)  [unwired: 1 in]
        n79 = Bundle By Name(cluster=w267, "Type"=w266, "Ctl Refnum"=w265) -> (w264:T9)
        n80 = call "Queue Driver.vi"("Queue In"=w270, "State[]"=string[] ["Scale Channel", "Update User Interface", "Save Runtime Info", "CheckForUnsavedChanges"], "error in (no error)"=w269, "Operation"=Operation."Enqueue N Elements without Data") -> ("error out"=w268:errorcluster)  [unwired: 8 in, 3 out]
      }
      event "setDefault": Value Change {
        n81 = event-data() -> ("Type"=w275:T14, "CtlRef"=w274:refnum<vi>)  [unwired: 1 in]
        n82 = Bundle By Name(cluster=w276, "Type"=w275, "Ctl Refnum"=w274) -> (w273:T9)
        n83 = call "Queue Driver.vi"("Queue In"=w278, "State[]"=string[] ["Validate Default State", "Set Default", "Check Interface Type", "Update User Interface", "Save Runtime Info", "CheckForUnsavedChanges"], "error in (no error)"=w279, "Operation"=Operation."Enqueue N Elements without Data") -> ("error out"=w277:errorcluster)  [unwired: 8 in, 3 out]
      }
    }
    n84 = call "Producer Error source.vi"("error in"=w45, "Producer Error"=w42) -> ("error out"=w44:errorcluster, "String"=w41:string)  [unwired: 7 in]
    n85 = call-dynamic "Send Error.vi"("error in"=w44, "Process State"=w41, "Configuration Interface in"=w40) -> ("error out"=w43:errorcluster)  [unwired: 7 in, 1 out]
  }
  n86 = while {
    tunnel: w26 -> [w297]
    shift-right: [w290] -> w23
    shift-left: w24 -> [w301]
    tunnel: w36 -> [w299]
    shift-right: [w291] -> w17
    shift-left: w3 -> [w298]
    stop <- w300 stop-if-true
    n87 = call "Queue Driver.vi"("Queue In"=w297, "error in (no error)"=w298, "Operation"=Operation."Dequeue") -> ("Queue Out"=w296:refnum<queue>, "State Out"=w295:string, "Data Out"=w294:variant, "error out"=w292:errorcluster)  [unwired: 9 in]
    n88 = case shown="\"Idle\", Default" w295 {
      selector: w295 -> [w310 w315 w328 w355 w360 w385 w422 w426 _ w550 w576 w597 w620 w674 w699 _ w748 w768 w779 w795 w802 w840 w884 w893 w909 w919 w947 w986 w1016 w1021 w1043]
      tunnel: w296 -> [_ _ _ _ _ _ _ _ w470 w525 w566 _ _ _ _ w706 _ _ _ _ w800 _ _ _ _ _ _ _ _ _ w1046]
      tunnel: w301 -> [w304 w312 w338 w357 w359 w389 w424 w446 w488 w538 w575 w596 w616 w670 w701 w703 w747 w766 w783 w797 w799 w839 w885 w890 w911 w926 w946 w997 w1018 w1034 w1048]
      tunnel: [w303 w311 w339 w357 w358 w386 w424 w445 w487 w536 w573 w595 w615 w669 w701 w702 w746 w765 w778 w797 w798 w838 w885 w889 w911 w923 w945 w995 w1018 w1034 w1048] -> w290
      tunnel: [_ _ _ _ _ _ _ _ _ _ _ _ _ _ _ _ _ _ _ _ _ _ _ _ _ _ _ _ _ _ TRUE] -> w300
      tunnel: w299 -> [_ _ _ _ _ _ _ _ _ _ _ _ _ _ _ _ _ _ _ _ _ _ _ _ _ _ _ _ w1020 w1036 _]
      tunnel: w292 -> [w308 w313 w337 w356 w362 w388 w423 w443 w475 w549 w562 w594 w619 w654 w700 w705 w728 w767 w781 w796 w801 w841 w883 w892 w910 w933 w949 w1002 w1017 w1024 w1044]
      tunnel: [w302 w314 w331 w356 w361 w387 w423 w447 w489 w528 w568 w593 w617 w665 w700 w707 w744 w769 w780 w796 w803 w842 w883 w886 w910 w912 w948 w992 w1019 w1029 w1047] -> w284
      tunnel: w294 -> [_ _ _ _ _ _ _ _ _ w548 w559 _ w618 w673 _ _ _ _ w782 _ _ _ _ _ _ _ _ _ _ _ _]
      tunnel: [w310 w315 w328 w355 w360 w385 w422 w426 "Activating Output Channel(s)" ("Error Location") w550 w576 w597 w620 w674 w699 "Set Default" w748 w768 w779 w795 w802 w840 w884 w893 w909 w919 w947 w986 w1016 w1021 w1043] -> w283
      frame "Idle", Default {
        # "Wait for user input"
        n89 = Unbundle By Name(w304) -> ("Current Config"=w309:refnum<class "Plugin_UI.lvclass">)
        n90 = property on="Property Node" class="Plugin_UI.lvclass"(reference=w309, error in=w308) -> (error out=w306:errorcluster, "Public:Module Configuration"=w307:refnum<class "Module Configuration.lvclass">)  [unwired: 1 out]
        n91 = property on="Property Node" class="Module Configuration.lvclass"(reference=w307, error in=w306) -> (error out=w302:errorcluster, "Public:Module Name"=w305:string)  [unwired: 1 out]
        n92 = Bundle By Name(cluster=w304, "Plugin Name"=w305) -> (w303:T11)
      }
      frame "Invoke Plugin" {
        # "Triggers when the plugin is selected in the Configuration tree"
        n93 = in-place "In Place Element Structure" {
          in-place-border: [w319] -> w314
          in-place-border: w313 -> [w318]
          n94 = in-place-cluster #1(w312) -> ("Current Config"=w317:refnum<class "Plugin_UI.lvclass">)
          n95 = call "Update Scaling Information.vi"("Plugin_UI in"=w317, "error in (no error)"=w318) -> ("Plugin_UI out"=w316:refnum<class "Plugin_UI.lvclass">, "error out"=w319:errorcluster)  [unwired: 12 in]
          n96 = in-place-cluster #1("Current Config"=w316) -> (w311:T11)
        }
      }
      frame "Initialize UI" {
        # "#PluginSpecificEdits_UI_10\nGet HW settings According to the Available Interface type"
        # "Read the latest details from Module Configuration"
        n97 = Unbundle By Name(w338) -> ("Default Ch. Status"=w334:bool, "Current Config"=w340:refnum<class "Plugin_UI.lvclass">)
        n98 = property on="Test Result" class="MCListbox (strict)"(error in=w337, "ItemNames"=string[][] [] ("Item Names")) -> (error out=w336:errorcluster)  [unwired: 1 in, 1 out]
        n99 = property on="Property Node" class="Plugin_UI.lvclass"(reference=w340, error in=w336) -> (reference out=w344:refnum<class "Plugin_UI.lvclass">, error out=w326:errorcluster, "Public:Module Configuration"=w327:refnum<class "Module Configuration.lvclass">)
        n100 = property on="Property Node" class="Module Configuration.lvclass"(reference=w327, error in=w326) -> (reference out=w325:refnum<class "Module Configuration.lvclass">, error out=w324:errorcluster, "Public:Lookup Tables"=w323:T20[], "Public:Scaling Functions"=w322:T21[])
        n101 = disable-structure "Diagram Disable Structure" shown="Disabled" {
          disable-tunnel: [w349 w351] -> w343
          disable-tunnel: [w348 w354] -> w342
          disable-tunnel: w325 -> [w347 w352]
          disable-tunnel: w324 -> [w346 w353]
          disable-tunnel: [w345 _] -> w321
          disable-tunnel: [_ w350] -> w320
          frame Disabled {
            n102 = call "Get UDP Settings.vi"("error in (no error)"=w346, "Module Configuration"=w347) -> ("error out"=w348:errorcluster, "UDP configuration"=w345:T23, "Module Configuration out"=w349:refnum<class "Module Configuration.lvclass">)  [unwired: 7 in]
          }
          frame Enabled {
            n103 = call "Get Serial Settings.vi"("error IO"=w353, "Module Configuration in"=w352) -> ("error IO Out"=w354:errorcluster, "Serial Configuration"=w350:T24, "Module Configuration out"=w351:refnum<class "Module Configuration.lvclass">)  [unwired: 7 in]
          }
        }
        n104 = call "Get All Channels.vi"("error in (no error)"=w342, "Default Channel Status"=w334, "Module Configuration"=w343) -> ("error out"=w330:errorcluster, "Output Channels[]"=w332:refnum<class "Output Channels.lvclass">[], "Input Channels[]"=w333:refnum<class "Input Channels.lvclass">[], "Module Configuration out"=w329:refnum<class "Module Configuration.lvclass">)  [unwired: 4 in, 1 out]
        n105 = property on="Property Node" class="Plugin_UI.lvclass"(reference=w344, error in=w330, "Public:Module Configuration"=w329, "Public:Input Channels[]"=w333, "Public:Output Channels[]"=w332, "Public:UDP Configuration"=w321, "Public:Serial Configuration"=w320, "private:Lookup Tables"=w323, "private:Scaling Functions"=w322) -> (reference out=w335:refnum<class "Plugin_UI.lvclass">, error out=w331:errorcluster)
        n106 = Bundle By Name(cluster=w338, "Current Config"=w335, "Initial Config"=w335) -> (w339:T11)
      }
      frame "------------Interface Page------------" {
      }
      frame "Update Hardware Configuration" {
        # "Update the changes in Hardware Configuration"
        n107 = in-place "In Place Element Structure" {
          in-place-border: w362 -> [w372]
          in-place-border: [w371] -> w361
          # "#PluginSpecificEdits_UI_9\n1. Enable the Serial setting or UDP (Required Settings) and Remove the Diagram Disble structure."
          n108 = in-place-cluster #2(w359) -> ("Current Config"=w364:refnum<class "Plugin_UI.lvclass">)
          n109 = property on="Property Node" class="Plugin_UI.lvclass"(reference=w364, error in=w372) -> (reference out=w369:refnum<class "Plugin_UI.lvclass">, error out=w370:errorcluster, "Public:UDP Configuration"=w368:T23, "Public:Serial Configuration"=w366:T24)
          n110 = disable-structure "Diagram Disable Structure" shown="Enabled" {
            disable-tunnel: w368 -> [w376 _]
            disable-tunnel: [w375 _] -> w367
            disable-tunnel: w366 -> [_ w382]
            disable-tunnel: [_ w381] -> w365
            frame Disabled {
              # "UDP Setting"
              n111 = Bundle By Name(cluster=w376, "Device IP"="Device IP", "Timeout"="Timeout (ms)") -> (w375:T23)
            }
            frame Enabled {
              # "Serial Settings"
              n112 = case shown="\"Invalid\", Default" "Interface Type" {
                tunnel: [w383 w384] -> w380
                frame "Invalid", Default {
                  w383 = T25 0 items=["GPIB"=1, "VXI"=2, "GPIB-VXI"=3, "Serial"=4, "PXI"=5, "TCPIP"=6, "USB"=7, "FireWire"=9, "Invalid"=0] ("Interface Type")
                }
                frame "Serial" {
                  w384 = T25 4 items=["GPIB"=1, "VXI"=2, "GPIB-VXI"=3, "Serial"=4, "PXI"=5, "TCPIP"=6, "USB"=7, "FireWire"=9, "Invalid"=0] ("Interface Type")
                }
              }
              n113 = Bundle By Name(cluster=w382, "VISA"="VISA", "Serial Interface"="Serial Interface", "Interface Type"=w380) -> (w381:T24)
            }
          }
          n114 = property on="Property Node" class="Plugin_UI.lvclass"(reference=w369, error in=w370, "Public:UDP Configuration"=w367, "Public:Serial Configuration"=w365) -> (reference out=w363:refnum<class "Plugin_UI.lvclass">, error out=w371:errorcluster)
          n115 = in-place-cluster #2("Current Config"=w363) -> (w358:T11)
        }
      }
      frame "Check Interface Type" {
        # "Read the interface type and update"
        n116 = in-place "In Place Element Structure" {
          in-place-border: w388 -> [w406]
          in-place-border: [w394] -> w387
          # "#PluginSpecificEdits_UI_17  Delete this case if the HW is UDP"
          n117 = in-place-cluster #3(w389) -> ("Current Config"=w405:refnum<class "Plugin_UI.lvclass">)
          n118 = property on="Property Node" class="Plugin_UI.lvclass"(reference=w405, error in=w406) -> (reference out=w397:refnum<class "Plugin_UI.lvclass">, error out=w404:errorcluster, "Public:Serial Configuration"=w399:T24)
          n119 = Unbundle By Name(w399) -> ("Interface Type"=w401:T25, "VISA"=w403:refnum<visa-resource-name>)
          n120 = property on="Property Node" class="Instr"(reference=w403, error in=w404) -> (error out=w402:errorcluster, "Intf Type"=w400:u16)  [unwired: 1 out]
          n121 = case shown="Error" w402 {
            selector: w402 -> [w410 w418]
            tunnel: w401 -> [_ w416]
            tunnel: w400 -> [w407 _]
            tunnel: [w410 w414] -> w393
            tunnel: [w409 w413] -> w391
            tunnel: [FALSE TRUE] -> w390
            tunnel: [w407 w416] -> w398
            frame No Error {
              n122 = case shown="4" w407 {
                tunnel: [Settings_Container."Invalid" ("Interface Type") Settings_Container."Serial" ("Interface Type")] -> w409
                frame Default {
                }
                frame 4 {
                }
              }
            }
            frame Error {
              # "Clearing the following errors,\n-1073807343 => When no resource is selected in VISA control\n-1073807346 => When the specified resource is not present in the system"
              n123 = call <vilib>:"Clear Errors.vi"("error in (no error)"=w418, "specific error code to clear (0: all)"=-1073807343) -> ("error out"=w421:errorcluster)  [unwired: 4 in, 1 out]
              n124 = call <vilib>:"Clear Errors.vi"("error in (no error)"=w421, "specific error code to clear (0: all)"=-1073807346) -> ("error out"=w415:errorcluster)  [unwired: 4 in, 1 out]
              n125 = property on="Interface Type" class="TabCtl (strict)"(error in=w415) -> (error out=w414:errorcluster, "Value"=w413:T4)  [unwired: 1 in, 1 out]
            }
          }
          n126 = Bundle By Name(cluster=w399, "Interface Type"=w398) -> (w396:T24)
          n127 = property on="Interface Type" class="TabCtl (strict)"(error in=w393, "Value"=w391, "Page Labels Display Visible?"=w390, "Label.Visible"=w390) -> (error out=w392:errorcluster)  [unwired: 1 in, 1 out]
          n128 = property on="Property Node" class="Plugin_UI.lvclass"(reference=w397, error in=w392, "Public:Serial Configuration"=w396) -> (reference out=w395:refnum<class "Plugin_UI.lvclass">, error out=w394:errorcluster)
          n129 = in-place-cluster #3("Current Config"=w395) -> (w386:T11)
        }
      }
      frame "------------Channel Page------------" {
      }
      frame "Update Output Channel" {
        # "#PluginSpecificEdits_UI_19\nAdd or remove the  Output settings based on settings available"
        # "Update the Output Channel Details into the Output Channel Object"
        n130 = Unbundle By Name(w446) -> ("Output Status"=w433:bool, "Current Config"=w442:refnum<class "Plugin_UI.lvclass">, "Output Ch. Name"=w428:string)
        n131 = property on="Property Node" class="Plugin_UI.lvclass"(reference=w442, error in=w443) -> (reference out=w438:refnum<class "Plugin_UI.lvclass">, error out=w441:errorcluster, "Public:Module Configuration"=w439:refnum<class "Module Configuration.lvclass">)
        n132 = Unbundle By Name("Output Settings") -> ("Channel Name"=w429:string, "Enable Output"=w430:bool, "Unit"=w448:string, "Value"=w425:dbl)
        n133 = Build Array(w429) -> (w437:string[])
        n134 = Build Array(w428) -> (w427:string[])
        n135 = call "Channel reduancy check.vi"("Show Pop up"=TRUE, "Old Channel Name[]"=w427, "error in"=w441, "New Channel Name[]"=w437, "Module configuration in"=w439) -> ("error out"=w440:errorcluster, "Error message"=w432:string, "Channel Configuration Found(F)"=w436:bool)  [unwired: 3 in, 1 out]
        n136 = case "Invalid Channel Name?" shown="False" w436 {
          tunnel: w430 -> [_ w456]
          tunnel: w448 -> [_ w466]
          tunnel: [w450 w464] -> w447
          tunnel: [w454 w460] -> w444
          tunnel: w440 -> [w451 w459]
          tunnel: w438 -> [w454 w458]
          tunnel: w429 -> [_ w457]
          tunnel: w428 -> [w453 _]
          tunnel: [w453 w457] -> w435
          tunnel: [w452 w456] -> w434
          tunnel: w433 -> [w452 _]
          tunnel: w432 -> [_ _]
          tunnel: w425 -> [_ w455]
          frame True {
            # "If Channel name is not valid, then revert to the latest valid name that was configured"
            n137 = property on="Channel Name" class="Str"(error in=w451, "Value"=w453) -> (error out=w450:errorcluster)  [unwired: 1 in, 1 out]
          }
          frame False {
            # "Update the Output Channel Object with the latest Output Channel Settings"
            n138 = property on="Property Node" class="Plugin_UI.lvclass"(reference=w458, error in=w459) -> (reference out=w461:refnum<class "Plugin_UI.lvclass">, error out=w467:errorcluster, "Public:Output Channels[]"=w469:refnum<class "Output Channels.lvclass">[])
            n139 = Index Array(array=w469) -> (element=w468:refnum<class "Output Channels.lvclass">)  [unwired: 1 in]
            n140 = property on="Property Node" class="Output Channels.lvclass"(reference=w468, error in=w467, "Public:Alias"=w457, "Public:Channel Active"=w456, "Public:Unit"=w466, "Public:Value"=w455) -> (reference out=w463:refnum<class "Output Channels.lvclass">, error out=w465:errorcluster)
            n141 = Build Array(w463) -> (w462:refnum<class "Output Channels.lvclass">[])
            n142 = property on="Property Node" class="Plugin_UI.lvclass"(reference=w461, error in=w465, "Public:Output Channels[]"=w462) -> (reference out=w460:refnum<class "Plugin_UI.lvclass">, error out=w464:errorcluster)
          }
        }
        n143 = Bundle By Name(cluster=w446, "Output Status"=w434, "Output Ch. Name"=w435, "Current Config"=w444) -> (w445:T11)
      }
      frame "Enable/Disable Output Channels" {
        # "Update the enable/disable status of the output channel"
        n144 = Unbundle By Name(w488) -> ("Output Status"=w478:bool, "Current Config"=w485:refnum<class "Plugin_UI.lvclass">, "Output Ch. Name"=w473:string)
        n145 = property on="Enable Output" class="Bool (strict)"(error in=w475) -> (error out=w474:errorcluster, "Value"=w472:bool)  [unwired: 1 in, 1 out]
        n146 = property on="Property Node" class="Plugin_UI.lvclass"(reference=w485, error in=w474) -> (reference out=w481:refnum<class "Plugin_UI.lvclass">, error out=w484:errorcluster, "Public:Module Configuration"=w482:refnum<class "Module Configuration.lvclass">)
        n147 = case shown="True" w472 {
          selector: w472 -> [w493 w494]
          tunnel: w484 -> [w492 w502]
          tunnel: [w492 w501] -> w483
          tunnel: w482 -> [_ w500]
          tunnel: [FALSE ("Channel Configuration Found(F)") w498] -> w480
          tunnel: ["" ("Empty String Constant") w497] -> w477
          tunnel: w473 -> [_ w495]
          tunnel: [w493 w494] -> w471
          frame False {
          }
          frame True {
            n148 = Build Array(w495) -> (w499:string[])
            n149 = call "Channel reduancy check.vi"("Show Pop up"=FALSE, "error in"=w502, "New Channel Name[]"=w499, "Module configuration in"=w500) -> ("error out"=w501:errorcluster, "Error message"=w497:string, "Channel Configuration Found(F)"=w498:bool)  [unwired: 4 in, 1 out]
          }
        }
        n150 = case "Invalid Channel Name?" shown="True" w480 {
          tunnel: w471 -> [_ w513]
          tunnel: [w510 w520] -> w489
          tunnel: [w512 w516] -> w486
          tunnel: w483 -> [w505 w515]
          tunnel: w481 -> [w512 w514]
          tunnel: [w507 w513] -> w479
          tunnel: w478 -> [w507 _]
          tunnel: w477 -> [w509 _]
          tunnel: w470 -> [w503 _]
          frame True {
            # "#PluginSpecificEdits_UI_23\nIf error logic is implemented ,Give Plugin specific error code \n[check the link for the available error code range\n https://wiki.bsh-sdd.com/display/LABSYS/Custom+Error+Code ]\nWrite the actual Plugin Name instead of Plugin name in the error message\n#Tobedefined Once the custom error code is defined , update the same in wiki. \nFor example: https://wiki.bsh-sdd.com/display/LABSYS/Almemo"
            # "If Channel name is not valid, then do not activate the channel"
            n151 = call "Queue Driver.vi"("Queue In"=w503, "error in (no error)"=w505, "Operation"=Operation."Flush") -> ("error out"=w504:errorcluster)  [unwired: 9 in, 3 out]
            n152 = property on="Enable Output" class="Bool (strict)"(error in=w504, "Value"=w507) -> (error out=w508:errorcluster)  [unwired: 1 in, 1 out]
            n153 = call <vilib>:"Error Cluster From Error Code.vi"("error in (no error)"=w508, "error message (\"\")"=w509, "error code (0)"=0) -> ("error out"=w510:errorcluster)  [unwired: 6 in]
          }
          frame False {
            # "Update the Output Channel Object with the latest Output Channel Settings"
            n154 = property on="Property Node" class="Plugin_UI.lvclass"(reference=w514, error in=w515) -> (reference out=w517:refnum<class "Plugin_UI.lvclass">, error out=w522:errorcluster, "Public:Output Channels[]"=w524:refnum<class "Output Channels.lvclass">[])
            n155 = Index Array(array=w524) -> (element=w523:refnum<class "Output Channels.lvclass">)  [unwired: 1 in]
            n156 = property on="Property Node" class="Output Channels.lvclass"(reference=w523, error in=w522, "Public:Channel Active"=w513) -> (reference out=w519:refnum<class "Output Channels.lvclass">, error out=w521:errorcluster)
            n157 = Build Array(w519) -> (w518:refnum<class "Output Channels.lvclass">[])
            n158 = property on="Property Node" class="Plugin_UI.lvclass"(reference=w517, error in=w521, "Public:Output Channels[]"=w518) -> (reference out=w516:refnum<class "Plugin_UI.lvclass">, error out=w520:errorcluster)
          }
        }
        n159 = Bundle By Name(cluster=w488, "Output Status"=w479, "Current Config"=w486) -> (w487:T11)
      }
      frame "Enable/Disable Input Channels" {
        w532 = TRUE  # Single Channel?
        w541 = 38
        n160 = Variant To Data(error in=w549, type=T16 {"Row"=0, "Column"=0} ("Edit Position"), Variant=w548) -> (data=w545:T16, error out=w546:errorcluster)
        n161 = Unbundle By Name(w545) -> ("Row"=w534:i32)
        n162 = property on="Measurement Channels" class="MCListbox (strict)"(error in=w546) -> (error out=w530:errorcluster, "ItemSyms"=w544:i32[])  [unwired: 1 in, 1 out]
        n163 = Index Array(array=w544, index=w534) -> (element=w543:i32)
        n164 = Equal?(x=w543, y=w541) -> (x = y?=w539:bool)
        n165 = Select(t=37, s=w539, f=w541) -> (s? t:f=w540:i32)
        n166 = Unbundle By Name(w538) -> ("Input Ch. Name[]"=w531:string[], "Current Config"=w533:refnum<class "Plugin_UI.lvclass">)
        n167 = Replace Array Subset(array=w544, new element=w540, index=w534) -> (w527:i32[])
        n168 = Not(x=w539) -> (.not. x?=w535:bool)
        n169 = call "Update Input Channel Active Status.vi"("Channel Index"=w534, "Input Ch. Name[]"=w531, "error in (no error)"=w530, "Activate Channel?"=w535, "Single Channel?"=w532, "Plugin_UI in"=w533) -> ("error out"=w529:errorcluster, "Error?"=w526:bool, "Plugin_UI out"=w537:refnum<class "Plugin_UI.lvclass">)  [unwired: 3 in]
        n170 = Bundle By Name(cluster=w538, "Current Config"=w537) -> (w536:T11)
        n171 = case "Error in Operation?" shown="False" w526 {
          tunnel: w529 -> [w553 w557]
          tunnel: [w552 w556] -> w528
          tunnel: w527 -> [w551 _]
          tunnel: w525 -> [_ w555]
          frame False {
            n172 = property on="Measurement Channels" class="MCListbox (strict)"(error in=w553, "ItemSyms"=w551) -> (error out=w552:errorcluster)  [unwired: 1 in, 1 out]
          }
          frame True {
            n173 = call "Queue Driver.vi"("Queue In"=w555, "error in (no error)"=w557, "Operation"=Operation."Flush") -> ("error out"=w556:errorcluster)  [unwired: 9 in, 3 out]
          }
        }
      }
      frame "Enable/Disable All Input Channels" {
        w571 = FALSE  # Single Channel?
        # "Enable or Disable All the Input Channels based on the Select All Value"
        n174 = Variant To Data(error in=w562, type=enum8{"False", "True", "Mixed"}."False" ("y"), Variant=w559) -> (data=w558:enum8{"False", "True", "Mixed"}, error out=w561:errorcluster)
        n175 = Unbundle By Name(w575) -> ("Input Ch. Name[]"=w570:string[], "Current Config"=w572:refnum<class "Plugin_UI.lvclass">)
        n176 = Equal?(x="Select All?", y=enum8{"False", "True", "Mixed"}."True") -> (x = y?=w563:bool)
        n177 = call "Update Input Channel Active Status.vi"("Input Ch. Name[]"=w570, "error in (no error)"=w561, "Activate Channel?"=w563, "Single Channel?"=w571, "Plugin_UI in"=w572) -> ("error out"=w569:errorcluster, "Error?"=w567:bool, "Plugin_UI out"=w574:refnum<class "Plugin_UI.lvclass">)  [unwired: 4 in]
        n178 = Bundle By Name(cluster=w575, "Current Config"=w574) -> (w573:T11)
        n179 = case "Error in Operation?" shown="True" w567 {
          tunnel: w569 -> [w584 w589]
          tunnel: [w583 w588] -> w568
          tunnel: w566 -> [_ w587]
          tunnel: w563 -> [w580 _]
          tunnel: w558 -> [_ w585]
          frame False {
            n180 = Select(t=38, s=w580, f=37) -> (s? t:f=w582:i32)
            n181 = Initialize Array(w582, 15 ("dimension size")) -> (w577:i32[])
            n182 = property on="Measurement Channels" class="MCListbox (strict)"(error in=w584, "ItemSyms"=w577) -> (error out=w583:errorcluster)  [unwired: 1 in, 1 out]
          }
          frame True {
            n183 = local write "Select All?"(w585) -> ()
            n184 = call "Queue Driver.vi"("Queue In"=w587, "error in (no error)"=w589, "Operation"=Operation."Flush") -> ("error out"=w588:errorcluster)  [unwired: 9 in, 3 out]
          }
        }
      }
      frame "Update Refresh Time" {
        # "Updates Refresh time in all the input channels"
        n185 = Unbundle By Name(w596) -> ("No. of Input Ch."=w590:i32, "Current Config"=w591:refnum<class "Plugin_UI.lvclass">)
        n186 = in-place "In Place Element Structure" {
          in-place-border: w594 -> [w600]
          in-place-border: [w603] -> w593
          in-place-border: w590 -> [w598]
          n187 = in-place-cluster #4(w591) -> ("Input Channels[]"=w602:refnum<class "Input Channels.lvclass">[])
          n188 = for {
            N: w598 -> [_]
            shift-right: [w606] -> w601
            shift-left: w602 -> [w609]
            shift-right: [w605] -> w603
            shift-left: w600 -> [w607]
            tunnel: "Refresh Time (ms)" -> [w604]
            i -> [w608]
            n189 = in-place "In Place Element Structure" {
              in-place-border: w607 -> [w613]
              in-place-border: [w611] -> w605
              in-place-border: w604 -> [w610]
              n190 = in-place-array #5(w609, w608) -> (w614:refnum<class "Input Channels.lvclass">)
              n191 = property on="Property Node" class="Input Channels.lvclass"(reference=w614, error in=w613, "Public:Refresh (ms)"=w610) -> (reference out=w612:refnum<class "Input Channels.lvclass">, error out=w611:errorcluster)
              n192 = in-place-array #5(w612) -> (w606:refnum<class "Input Channels.lvclass">[])  [unwired: 1 out]
            }
          }
          n193 = in-place-cluster #4("Input Channels[]"=w601) -> (w592:refnum<class "Plugin_UI.lvclass">)
        }
        n194 = Bundle By Name(cluster=w596, "Current Config"=w592) -> (w595:T11)
      }
      frame "Update Channel Unit" {
        # "Read the new Unit & update in the corresponding Channel Object"
        n195 = in-place "In Place Element Structure" {
          in-place-border: w619 -> [w638]
          in-place-border: w618 -> [w637]
          in-place-border: [w625] -> w617
          n196 = in-place-cluster #6(w616) -> ("Current Config"=w622:refnum<class "Plugin_UI.lvclass">)
          n197 = Variant To Data(error in=w638, type=T16 {"Row"=0, "Column"=0} ("Edit Position"), Variant=w637) -> (data=w634:T16, error out=w635:errorcluster)
          n198 = property on="Measurement Channels" class="MCListbox (strict)"(error in=w635) -> (error out=w631:errorcluster, "ItemNames"=w633:string[][])  [unwired: 1 in, 1 out]
          n199 = Unbundle By Name(w634) -> ("Row"=w629:i32)
          n200 = property on="Property Node" class="Plugin_UI.lvclass"(reference=w622, error in=w631) -> (reference out=w623:refnum<class "Plugin_UI.lvclass">, error out=w627:errorcluster, "Public:Input Channels[]"=w630:refnum<class "Input Channels.lvclass">[])
          n201 = Index Array(array=w633, index (row)=w629, index (col)=2 ("disabled index (col)")) -> (element=w628:string)
          n202 = in-place "In Place Element Structure" {
            in-place-border: w628 -> [w642]
            in-place-border: w627 -> [w646]
            in-place-border: [w640] -> w626
            n203 = in-place-array #7(w630, w629) -> (w647:refnum<class "Input Channels.lvclass">)
            n204 = property on="Property Node" class="Input Channels.lvclass"(reference=w647, error in=w646) -> (reference out=w643:refnum<class "Input Channels.lvclass">, error out=w644:errorcluster, "Public:Scaling Information"=w645:T26)
            n205 = Bundle By Name(cluster=w645, "Output Unit"=w642) -> (w641:T26)
            n206 = property on="Property Node" class="Input Channels.lvclass"(reference=w643, error in=w644, "Public:Scaling Information"=w641) -> (reference out=w639:refnum<class "Input Channels.lvclass">, error out=w640:errorcluster)
            n207 = in-place-array #7(w639) -> (w624:refnum<class "Input Channels.lvclass">[])  [unwired: 1 out]
          }
          n208 = property on="Property Node" class="Plugin_UI.lvclass"(reference=w623, error in=w626, "Public:Input Channels[]"=w624) -> (reference out=w621:refnum<class "Plugin_UI.lvclass">, error out=w625:errorcluster)
          n209 = in-place-cluster #6("Current Config"=w621) -> (w615:T11)
        }
      }
      frame "Update Channel Name" {
        # "Read the new Channel Name & update in the corresponding Channel Object"
        n210 = property on="Measurement Channels" class="MCListbox (strict)"(error in=w654) -> (error out=w653:errorcluster, "ItemNames"=w650:string[][])  [unwired: 1 in, 1 out]
        n211 = Unbundle By Name(w670) -> ("Current Config"=w667:refnum<class "Plugin_UI.lvclass">, "Input Ch. Name[]"=w649:string[])
        n212 = Variant To Data(error in=w653, type=T16 {"Row"=0, "Column"=0} ("Edit Position"), Variant=w673) -> (data=w671:T16, error out=w652:errorcluster)
        n213 = Unbundle(w671) -> ("Row"=w656:i32)  [unwired: 1 out]
        n214 = Index Array(array=w649, index=w656) -> (element=w655:string)
        n215 = Index Array(array=w650, index (row)=w656, index (col)=1 ("disabled index (col)")) -> (element=w657:string)
        n216 = property on="Property Node" class="Plugin_UI.lvclass"(reference=w667, error in=w652) -> (reference out=w663:refnum<class "Plugin_UI.lvclass">, error out=w660:errorcluster, "Public:Module Configuration"=w658:refnum<class "Module Configuration.lvclass">, "Public:Input Channels[]"=w666:refnum<class "Input Channels.lvclass">[])
        n217 = Build Array(w657) -> (w661:string[])
        n218 = Build Array(w655) -> (w662:string[])
        n219 = call "Channel reduancy check.vi"("Old Channel Name[]"=w662, "error in"=w660, "New Channel Name[]"=w661, "Module configuration in"=w658) -> ("error out"=w659:errorcluster, "Channel Configuration Found(F)"=w651:bool)  [unwired: 4 in, 2 out]
        n220 = case "Invalid Channel Name?" shown="False" w651 {
          tunnel: w666 -> [w686 _]
          tunnel: [w684 w696] -> w665
          tunnel: [w683 w698] -> w664
          tunnel: w663 -> [w681 w698]
          tunnel: w659 -> [w680 w697]
          tunnel: w657 -> [w679 _]
          tunnel: w656 -> [w678 _]
          tunnel: w650 -> [w677 w695]
          tunnel: w649 -> [_ w692]
          tunnel: [w675 w692] -> w648
          frame False {
            # "Update the Input Channel Object with the latest Input Channel Name"
            n221 = in-place "In Place Element Structure" {
              in-place-border: w680 -> [w689]
              in-place-border: [w691] -> w685
              in-place-border: w679 -> [w687]
              n222 = in-place-array #8(w686, w678) -> (w688:refnum<class "Input Channels.lvclass">)
              n223 = property on="Property Node" class="Input Channels.lvclass"(reference=w688, error in=w689, "Public:Alias"=w687) -> (reference out=w690:refnum<class "Input Channels.lvclass">, error out=w691:errorcluster)
              n224 = in-place-array #8(w690) -> (w682:refnum<class "Input Channels.lvclass">[])  [unwired: 1 out]
            }
            n225 = Index Array(array=w677, index (col)=1 ("disabled index (col)")) -> (element=w675:string[])  [unwired: 1 in]
            n226 = property on="Property Node" class="Plugin_UI.lvclass"(reference=w681, error in=w685, "Public:Input Channels[]"=w682) -> (reference out=w683:refnum<class "Plugin_UI.lvclass">, error out=w684:errorcluster)
          }
          frame True {
            # "If Channel name is not valid, then revert to the latest valid name that was configured"
            n227 = Replace Array Subset(array=w695, new element=w692, index (col)=1 ("disabled index (col)")) -> (w694:string[][])  [unwired: 1 in]
            n228 = property on="Measurement Channels" class="MCListbox (strict)"(error in=w697, "ItemNames"=w694) -> (error out=w696:errorcluster)  [unwired: 1 in, 1 out]
          }
        }
        n229 = Bundle By Name(cluster=w670, "Current Config"=w664, "Input Ch. Name[]"=w648) -> (w669:T11)
      }
      frame "------------Toolbar------------" {
      }
      frame "Validate Default State" {
        # "#PluginSpecificEdits_UI_21\nIf error logic is implemented ,Give Plugin specific error code [check the link for the available error code range https://wiki.bsh-sdd.com/display/LABSYS/Custom+Error+Code ]\nWrite the actual Plugin Name instead of Plugin name in the error message\n#Tobedefined Once the custom error code is defined , update the same in wiki. For example: https://wiki.bsh-sdd.com/display/LABSYS/Almemo"
        # "This case checks if the Channel names in Init Config is valid of not. If there is any issues, generates an error and discard the Set Default action"
        n230 = in-place "In Place Element Structure" {
          in-place-border: [w712] -> w707
          in-place-border: w706 -> [w711]
          in-place-border: w705 -> [w710]
          n231 = in-place-cluster #9(w703) -> ("Initial Config"=w709:refnum<class "Plugin_UI.lvclass">)
          n232 = call "Validate Default State.vi"("error in (no error)"=w710, "Plugin_UI in"=w709) -> ("error out"=w715:errorcluster, "Error message"=w713:string, "Conflicts in Default State?"=w714:bool, "Plugin_UI out"=w708:refnum<class "Plugin_UI.lvclass">)  [unwired: 6 in]
          n233 = case shown="True" w714 {
            tunnel: w715 -> [w716 w721]
            tunnel: w713 -> [_ w723]
            tunnel: [w716 w719] -> w712
            tunnel: w711 -> [_ w718]
            frame False {
            }
            frame True {
              n234 = call "Queue Driver.vi"("Queue In"=w718, "error in (no error)"=w721, "Operation"=Operation."Flush") -> ("error out"=w720:errorcluster)  [unwired: 9 in, 3 out]
              n235 = call <vilib>:"Error Cluster From Error Code.vi"("error in (no error)"=w720, "error message (\"\")"=w723, "error code (0)"=0) -> ("error out"=w719:errorcluster)  [unwired: 6 in]
            }
          }
          n236 = in-place-cluster #9("Initial Config"=w708) -> (w702:T11)
        }
      }
      frame "Set Default" {
        # "Set Current Config to default state and disables the Set default button"
        n237 = property on="Test Result" class="MCListbox (strict)"(error in=w728, "ItemNames"=string[][] [] ("Item Names")) -> (error out=w724:errorcluster, "NumRows"=w725:u32)  [unwired: 1 in, 1 out]
        n238 = To Long Integer(number=w725) -> (32bit integer=w729:i32)
        n239 = for {
          N: w729 -> [_]
          tunnel: T16 {"Row"=0, "Column"=4} ("Active Cell:Active Cell") -> [w752]
          tunnel: u32 16448250 ("Color Box") -> [w751]
          shift-right: [w749] -> w727
          shift-left: w724 -> [w750]
          i -> [w754]
          n240 = Bundle By Name(cluster=w752, "Row"=w754) -> (w753:T16)
          n241 = property on="Test Result" class="MCListbox (strict)"(error in=w750, "ActiveCell"=w753, "CellBG"=w751) -> (error out=w749:errorcluster)  [unwired: 1 in, 1 out]
        }
        n242 = Unbundle By Name(w747) -> ("Initial Config"=w743:refnum<class "Plugin_UI.lvclass">)
        n243 = property on="Property Node" class="Plugin_UI.lvclass"(reference=w743, error in=w727) -> (reference out=w735:refnum<class "Plugin_UI.lvclass">, error out=w740:errorcluster, "Public:Module Configuration"=w742:refnum<class "Module Configuration.lvclass">, "private:Lookup Tables"=w741:T20[], "private:Scaling Functions"=w738:T21[])
        n244 = for {
          shift-right: [w758] -> w739
          shift-left: w740 -> [w759]
          shift-right: [w757] -> w737
          shift-left: w742 -> [w756]
          tunnel: w741 -> [w755] mode=indexing
          n245 = call "Set Lookup Table.vi"("error in (no error)"=w759, "Table Information"=w755, "Module Configuration in"=w756) -> ("error out"=w758:errorcluster, "Module Configuration out"=w757:refnum<class "Module Configuration.lvclass">)  [unwired: 7 in]
        }
        n246 = for {
          shift-right: [w760] -> w736
          shift-left: w739 -> [w763]
          shift-right: [w761] -> w733
          shift-left: w737 -> [w764]
          tunnel: w738 -> [w762] mode=indexing
          n247 = call "Set Scaling Function.vi"("error in (no error)"=w763, "Function Information"=w762, "Module Configuration in"=w764) -> ("error out"=w760:errorcluster, "Module Configuration out"=w761:refnum<class "Module Configuration.lvclass">)  [unwired: 7 in]
        }
        n248 = property on="Property Node" class="Plugin_UI.lvclass"(reference=w735, error in=w736, "Public:Module Configuration"=w733) -> (reference out=w732:refnum<class "Plugin_UI.lvclass">, error out=w734:errorcluster)
        n249 = Bundle By Name(cluster=w747, "Initial Config"=w732, "Current Config"=w732) -> (w746:T11)
        n250 = property on="setDefault" class="Bool (strict)"(error in=w734, "DisabledEnum"=T19."Disabled and Grayed Out" ("Disabled")) -> (error out=w744:errorcluster)  [unwired: 1 in, 1 out]
      }
      frame "Scale Channel" {
        n251 = in-place "In Place Element Structure" {
          in-place-border: [w777] -> w769
          in-place-border: w767 -> [w774]
          n252 = in-place-cluster #10(w766) -> ("Current Config"=w776:refnum<class "Plugin_UI.lvclass">, "Input Ch. Name[]"=w773:string[])
          n253 = property on="Measurement Channels" class="MCListbox (strict)"(error in=w774) -> (error out=w771:errorcluster, "Value"=w772:i32)  [unwired: 1 in, 1 out]
          n254 = Index Array(array=w773, index=w772) -> (element=w770:string)
          n255 = call "Configure Scaling.vi"("Plugin_UI in"=w776, "error in (no error)"=w771, "Selected Channel"=w770) -> ("Plugin_UI out"=w775:refnum<class "Plugin_UI.lvclass">, "error out"=w777:errorcluster)  [unwired: 10 in, 1 out]
          n256 = in-place-cluster #10("Current Config"=w775, "Input Ch. Name[]"=w773) -> (w765:T11)
        }
      }
      frame "ScalingEnabled?" {
        # "Enbale/Disable Scaling Button"
        n257 = in-place "In Place Element Structure" {
          in-place-border: w782 -> [w790]
          in-place-border: w781 -> [w789]
          in-place-border: [w786] -> w780
          n258 = in-place-cluster #11(w783) -> ("Current Config"=w785:refnum<class "Plugin_UI.lvclass">, "Initial Config"=w784:refnum<class "Plugin_UI.lvclass">)
          n259 = Variant To Data(error in=w789, type=TRUE, Variant=w790) -> (data=w792:bool, error out=w791:errorcluster)
          n260 = property on="Property Node" class="Plugin_UI.lvclass"(reference=w785, error in=w791, "Public:ScalingEnabled?"=w792) -> (reference out=w788:refnum<class "Plugin_UI.lvclass">, error out=w794:errorcluster)
          n261 = property on="Property Node" class="Plugin_UI.lvclass"(reference=w784, error in=w794, "Public:ScalingEnabled?"=w792) -> (reference out=w787:refnum<class "Plugin_UI.lvclass">, error out=w786:errorcluster)
          n262 = in-place-cluster #11("Current Config"=w788, "Initial Config"=w787) -> (w778:T11)
        }
      }
      frame "------------Test Page------------" {
      }
      frame "Consistency Check" {
        # "#PluginSpecificEdits_UI_30\nIf error logic is implemented ,Give Plugin specific error code [check the link for the available error code range https://wiki.bsh-sdd.com/display/LABSYS/Custom+Error+Code ]\nWrite the actual Plugin Name instead of Plugin name in the error message\n#Tobedefined Once the custom error code is defined , update the same in wiki. For example: https://wiki.bsh-sdd.com/display/LABSYS/Almemo"
        n263 = in-place "In Place Element Structure" {
          in-place-border: [w811] -> w803
          in-place-border: w801 -> [w810]
          in-place-border: w800 -> [w806]
          n264 = in-place-cluster #12(w799) -> ("Current Config"=w805:refnum<class "Plugin_UI.lvclass">)
          n265 = call "Initialize Controller Class.vi"("Plugin_UI in"=w805, "error in (no error)"=w810) -> ("Plugin_UI Out"=w807:refnum<class "Plugin_UI.lvclass">, "Plugin_Controller out"=w808:refnum<class "Plugin_Controller.lvclass">, "error out"=w809:errorcluster)  [unwired: 11 in]
          n266 = call-dynamic "Check Consistency.vi"("error in"=w809, "Plugin_Controller in"=w808) -> ("error out"=w814:errorcluster, "Result Messages"=w812:T28[], "Node OK"=w813:bool)  [unwired: 6 in, 1 out]
          n267 = case shown="False" w813 {
            tunnel: w807 -> [w826 w837]
            tunnel: [w826 w837] -> w804
            tunnel: w814 -> [w821 w836]
            tunnel: [w815 w836] -> w811
            tunnel: w812 -> [w822 _]
            tunnel: w806 -> [w820 _]
            frame False {
              n268 = for {
                tunnel: w822 -> [w835] mode=indexing
                tunnel: [w834] -> w823 mode=indexing
                n269 = Unbundle By Name(w835) -> ("Explanation"=w834:string)
              }
              n270 = Array To Spreadsheet String(delimiter (Tab)="\r\n" ("End of Line Constant"), array=w823, 3:"%s" ("format string")) -> (spreadsheet string=w817:string)
              n271 = call "Queue Driver.vi"("Queue In"=w820, "error in (no error)"=w821, "Operation"=Operation."Flush") -> ("error out"=w816:errorcluster)  [unwired: 9 in, 3 out]
              n272 = xnode ("Error Ring")("parameter 0"=w817) -> ("error out"=w818:errorcluster)
              n273 = Merge Errors(w816, w818) -> (w815:errorcluster)
            }
            frame True {
            }
          }
          n274 = in-place-cluster #12("Current Config"=w804) -> (w798:T11)
        }
      }
      frame "Test" {
        # "Test the current configuration"
        n275 = in-place "In Place Element Structure" {
          in-place-border: [w854] -> w842
          in-place-border: w841 -> [w865]
          # "#PluginSpecificEdits_UI_29 No of output channels"
          n276 = in-place-cluster #13(w839) -> ("Current Config"=w857:refnum<class "Plugin_UI.lvclass">, "No. of Input Ch."=w852:i32)
          n277 = call "SetCursorBusy.vi"("error in (no error)"=w865) -> ("error out"=w864:errorcluster)  [unwired: 10 in]
          n278 = property on="Test Result" class="MCListbox (strict)"(error in=w864, "ItemNames"=string[][] [] ("Item Names")) -> (error out=w866:errorcluster)  [unwired: 1 in, 1 out]
          n279 = Add(x=w852, y=0) -> (x+y=w850:i32)
          n280 = for {
            N: w850 -> [_]
            shift-right: [w871] -> w847
            shift-left: w866 -> [w873]
            tunnel: T16 {"Row"=0, "Column"=4} ("Active Cell:Active Cell") -> [w870]
            i -> [w869]
            n281 = Bundle By Name(cluster=w870, "Row"=w869) -> (w868:T16)
            n282 = property on="Test Result" class="MCListbox (strict)"(error in=w873, "ActiveCell"=w868, "CellBG"=u32 16448250 ("Color Box")) -> (error out=w871:errorcluster)  [unwired: 1 in, 1 out]
          }
          n283 = property on="Start Test" class="Bool"(error in=w847, "BoolText.Text"="Wait.." ("Boolean Text.Text")) -> (error out=w848:errorcluster)  [unwired: 1 in, 1 out]
          n284 = call "Run Test.vi"("error in (no error)"=w848, "Plugin_UI in"=w857) -> ("error out"=w859:errorcluster, "Plugin_Controller out"=w863:refnum<class "Plugin_Controller.lvclass">, "Plugin_UI out"=w856:refnum<class "Plugin_UI.lvclass">)  [unwired: 7 in]
          n285 = call "Eval Test.vi"("error in (no error)"=w859, "Plugin_Controller in"=w863) -> ("error out"=w861:errorcluster, "Passed?"=w862:bool[], "Result String"=w858:string[][])  [unwired: 6 in, 1 out]
          n286 = for {
            tunnel: w862 -> [w879] mode=indexing
            shift-right: [w876] -> w849
            shift-left: w861 -> [w875]
            tunnel: T16 {"Row"=0, "Column"=4} ("Active Cell:Active Cell") -> [w874]
            i -> [w880]
            n287 = Bundle By Name(cluster=w874, "Row"=w880) -> (w878:T16)
            n288 = Select(t=u32 6618880 ("Color Box"), s=w879, f=u32 16711680 ("Color Box")) -> (s? t:f=w877:u32)
            n289 = property on="Test Result" class="MCListbox (strict)"(error in=w875, "ActiveCell"=w878, "CellBG"=w877) -> (error out=w876:errorcluster)  [unwired: 1 in, 1 out]
          }
          n290 = property on="Test Result" class="MCListbox (strict)"(error in=w849, "ItemNames"=w858) -> (error out=w855:errorcluster)  [unwired: 1 in, 1 out]
          n291 = call "SetCursorFree.vi"("error in (no error)"=w855) -> ("error out"=w845:errorcluster)  [unwired: 10 in]
          n292 = property on="Start Test" class="Bool"(error in=w845, "BoolText.Text"="Test" ("Boolean Text.Text")) -> (error out=w844:errorcluster)  [unwired: 1 in, 1 out]
          n293 = in-place-cluster #13("Current Config"=w856, "No. of Input Ch."=w852) -> (w838:T11)
          n294 = Merge Errors(w844, w849) -> (w854:errorcluster)
        }
      }
      frame "-------------Metadata Informaton-----------" {
      }
      frame "Get Device Meta Data" {
        n295 = call "SetCursorBusy.vi"("error in (no error)"=w892) -> ("error out"=w891:errorcluster)  [unwired: 10 in]
        n296 = in-place "In Place Element Structure" {
          in-place-border: w891 -> [w906]
          in-place-border: [w896] -> w888
          n297 = in-place-cluster #14(w890) -> ("Current Config"=w905:refnum<class "Plugin_UI.lvclass">)
          n298 = call "Initialize Controller Class.vi"("Plugin_UI in"=w905, "error in (no error)"=w906) -> ("Plugin_UI Out"=w901:refnum<class "Plugin_UI.lvclass">, "Plugin_Controller out"=w904:refnum<class "Plugin_Controller.lvclass">, "error out"=w903:errorcluster)  [unwired: 11 in]
          n299 = call-dynamic "Init.vi"("error in"=w903, "Plugin_Controller in"=w904) -> ("error out"=w898:errorcluster, "Plugin_Controller out"=w902:refnum<class "Plugin_Controller.lvclass">)  [unwired: 8 in]
          n300 = flat-sequence {
            tunnel: w898 -> [w908]
            tunnel: [w908] -> w897
            frame #0 {
              n301 = Wait (ms)(milliseconds to wait=u32 500) -> ()  [unwired: 1 out]
            }
          }
          n302 = call-dynamic "DeInit.vi"("error in"=w897, "Plugin_Controller in"=w902) -> ("error out"=w900:errorcluster, "Plugin_Controller out"=w899:refnum<class "Plugin_Controller.lvclass">)  [unwired: 8 in]
          n303 = call "Evaluate Meta Data.vi"("error IO"=w900, "Plugin_Controller"=w899) -> ("error out"=w895:errorcluster, "Device Meta Data"=w894:T2)  [unwired: 8 in]
          n304 = property on="Device Meta Data" class="Clust"(error in=w895, "Value"=w894) -> (error out=w896:errorcluster)  [unwired: 1 in, 1 out]
          n305 = in-place-cluster #14("Current Config"=w901) -> (w889:T11)
        }
        n306 = call "SetCursorFree.vi"("error in (no error)"=w888) -> ("error out"=w887:errorcluster)  [unwired: 10 in]
        n307 = Merge Errors(w887, w888) -> (w886:errorcluster)
      }
      frame "------------Reusable Functions------------" {
      }
      frame "Update User Interface" {
        # "#PluginSpecificEdits_UI_8\n1. Used hardware configuration make Enable and \nRemove the Digram disable structure\n2. Update Hardware Configuration"
        # "#PluginSpecificEdits_UI_20\n\nUpdate the Output Setting\nUpdate required hardware settings \nand remove unused Hardware settings"
        # "Update the Interface & Channel Details in the UI"
        n308 = Unbundle By Name(w926) -> ("Current Config"=w934:refnum<class "Plugin_UI.lvclass">)
        n309 = property on="Property Node" class="Plugin_UI.lvclass"(reference=w934, error in=w933) -> (error out=w931:errorcluster, "Public:Output Channels[]"=w932:refnum<class "Output Channels.lvclass">[], "Public:Input Channels[]"=w918:refnum<class "Input Channels.lvclass">[], "Public:UDP Configuration"=w930:T23, "Public:Serial Configuration"=w913:T24)  [unwired: 1 out]
        n310 = disable-structure "Diagram Disable Structure" shown="Enabled" {
          disable-tunnel: w930 -> [w937 _]
          disable-tunnel: w913 -> [_ w942]
          frame Disabled {
            # "UDP"
            n311 = Unbundle By Name(w937) -> ("Device IP"=w936:string, "Timeout"=w935:i32)
            n312 = local write "Timeout (ms)"(w935) -> ()
            n313 = local write "Device IP"(w936) -> ()
          }
          frame Enabled {
            n314 = Unbundle By Name(w942) -> ("VISA"=w941:refnum<visa-resource-name>, "Serial Interface"=w940:T5, "Interface Type"=w939:T25)
            n315 = case shown="4" w939 {
              tunnel: [Settings_Container."Invalid" ("Interface Type") Settings_Container."Serial" ("Interface Type")] -> w938
              frame Default {
              }
              frame 4 {
              }
            }
            n316 = local write "VISA"(w941) -> ()
            n317 = local write "Serial Interface"(w940) -> ()
            n318 = local write "Interface Type"(w938) -> ()
          }
        }
        n319 = call "Get Output Channel.vi"("error in (no error)"=w931, "Output Channels[]"=w932) -> ("error out"=w914:errorcluster, "Output Channel Details"=w925:T6)  [unwired: 8 in]
        n320 = Unbundle By Name(w925) -> ("Enable Output"=w915:bool, "Channel Name"=w924:string)
        n321 = local write "Output Settings"(w925) -> ()
        n322 = call "Get Input Channel.vi"("Input Channels[]"=w918, "error in (no error)"=w914) -> ("Scale Active?"=w927:bool, "Input Channel Details[][]"=w922:string[][], "Channel Selection[]"=w928:i32[], "Select All"=w916:enum8{"False", "True", "Mixed"}, "Refresh (ms)"=w917:dbl, "error out"=w929:errorcluster)  [unwired: 7 in, 1 out]
        n323 = local write "scale"(w927) -> ()
        n324 = local write "Select All?"(w916) -> ()
        n325 = local write "Refresh Time (ms)"(w917) -> ()
        n326 = Index Array(array=w922, index (col)=1 ("disabled index (col)")) -> (element=w920:string[])  [unwired: 1 in]
        n327 = property on="Measurement Channels" class="MCListbox (strict)"(error in=w929, "ItemNames"=w922, "ItemSyms"=w928) -> (error out=w912:errorcluster)  [unwired: 1 in, 1 out]
        n328 = Bundle By Name(cluster=w926, "Output Status"=w915, "Output Ch. Name"=w924, "Input Ch. Name[]"=w920) -> (w923:T11)
      }
      frame "Save Runtime Info" {
        # "Save the content in Module Configuration"
        n329 = in-place "In Place Element Structure" {
          in-place-border: w949 -> [w969]
          in-place-border: [w966] -> w948
          # "#PluginSpecificEdits_UI_7\nDelete HW Settings\n2. Enable the \"SET UDP SETTING vi\" and Remove the Diagram Disble structure.\n(or)\n2. Enable the \"SET SERIAL SETTING vi\" and Remove the Diagram Disble structure."
          n330 = in-place-cluster #15(w946) -> ("Current Config"=w951:refnum<class "Plugin_UI.lvclass">)
          n331 = property on="Property Node" class="Plugin_UI.lvclass"(reference=w951, error in=w969) -> (reference out=w967:refnum<class "Plugin_UI.lvclass">, error out=w968:errorcluster, "Public:Module Configuration"=w972:refnum<class "Module Configuration.lvclass">, "Public:UDP Configuration"=w970:T23, "Public:Serial Configuration"=w952:T24, "Public:Input Channels[]"=w965:refnum<class "Input Channels.lvclass">[], "Public:Output Channels[]"=w964:refnum<class "Output Channels.lvclass">[], "private:Lookup Tables"=w954:T20[], "private:Scaling Functions"=w953:T21[])
          n332 = disable-structure "Diagram Disable Structure" shown="Disabled" {
            disable-tunnel: [w978 w983] -> w973
            disable-tunnel: w972 -> [w977 w981]
            disable-tunnel: [w976 w980] -> w971
            disable-tunnel: w970 -> [w975 _]
            disable-tunnel: w968 -> [w974 w982]
            disable-tunnel: w952 -> [_ w979]
            frame Disabled {
              n333 = call "Set UDP Settings.vi"("error in (no error)"=w974, "Hardware Configuration"=w975, "Module Configuration"=w977) -> ("error out"=w978:errorcluster, "Module Configuration out"=w976:refnum<class "Module Configuration.lvclass">)  [unwired: 7 in]
            }
            frame Enabled {
              n334 = call "Set Serial Settings.vi"("error IO"=w982, "Serial Configuration"=w979, "Module Configuration"=w981) -> ("error IO out"=w983:errorcluster, "Module Configuration out"=w980:refnum<class "Module Configuration.lvclass">)  [unwired: 7 in]
            }
          }
          n335 = Build Array (concatenate)(w965, w964) -> (w963:refnum<class "Plugin_Channels.lvclass">[])
          n336 = call "Set All Channels.vi"("error in"=w973, "Channels[]"=w963, "Module Configuration in"=w971) -> ("error out"=w962:errorcluster, "Module Configuration out"=w961:refnum<class "Module Configuration.lvclass">)  [unwired: 7 in]
          n337 = call "Set Value.vi"("error in (no error)"=w962, "Value"="Yes", "Key"="Saved Plugin", "Module Configuration in"=w961) -> ("error out"=w956:errorcluster, "Module Configuration out"=w958:refnum<class "Module Configuration.lvclass">)  [unwired: 6 in]
          n338 = property on="Property Node" class="Module Configuration.lvclass"(reference=w958, error in=w956, "Public:Lookup Tables"=w954, "Public:Scaling Functions"=w953) -> (reference out=w957:refnum<class "Module Configuration.lvclass">, error out=w955:errorcluster)
          n339 = property on="Property Node" class="Plugin_UI.lvclass"(reference=w967, error in=w955, "Public:Module Configuration"=w957) -> (reference out=w950:refnum<class "Plugin_UI.lvclass">, error out=w966:errorcluster)
          n340 = in-place-cluster #15("Current Config"=w950) -> (w945:T11)
        }
      }
      frame "Update Initial Config" {
        # "#PluginSpecificEdits_UI_6\nUpdate the HW Settings according to the available HW"
        # "This case will be executed once Save Configuration button is clicked"
        n341 = Unbundle By Name(w997) -> ("Current Config"=w998:refnum<class "Plugin_UI.lvclass">)
        n342 = property on="Property Node" class="Plugin_UI.lvclass"(reference=w998, error in=w1002) -> (reference out=w999:refnum<class "Plugin_UI.lvclass">, error out=w1001:errorcluster, "Public:Module Configuration"=w1004:refnum<class "Module Configuration.lvclass">, "Public:UDP Configuration"=w991:T23, "Public:Serial Configuration"=w984:T24, "Public:Input Channels[]"=w990:refnum<class "Input Channels.lvclass">[], "Public:Output Channels[]"=w989:refnum<class "Output Channels.lvclass">[])
        n343 = disable-structure "Diagram Disable Structure" shown="Disabled" {
          disable-tunnel: [w1010 w1014] -> w1005
          disable-tunnel: w1004 -> [w1009 w1013]
          disable-tunnel: w1001 -> [w1007 w1015]
          disable-tunnel: w991 -> [w1006 _]
          disable-tunnel: [w1008 w1012] -> w985
          disable-tunnel: w984 -> [_ w1011]
          frame Disabled {
            n344 = call "Set UDP Settings.vi"("error in (no error)"=w1007, "Hardware Configuration"=w1006, "Module Configuration"=w1009) -> ("error out"=w1010:errorcluster, "Module Configuration out"=w1008:refnum<class "Module Configuration.lvclass">)  [unwired: 7 in]
          }
          frame Enabled {
            n345 = call "Set Serial Settings.vi"("error IO"=w1015, "Serial Configuration"=w1011, "Module Configuration"=w1013) -> ("error IO out"=w1014:errorcluster, "Module Configuration out"=w1012:refnum<class "Module Configuration.lvclass">)  [unwired: 7 in]
          }
        }
        n346 = Build Array (concatenate)(w990, w989) -> (w988:refnum<class "Plugin_Channels.lvclass">[])
        n347 = call "Set All Channels.vi"("error in"=w1005, "Channels[]"=w988, "Module Configuration in"=w985) -> ("error out"=w1000:errorcluster, "Module Configuration out"=w1003:refnum<class "Module Configuration.lvclass">)  [unwired: 7 in]
        n348 = property on="Property Node" class="Plugin_UI.lvclass" props=["Public:Module Configuration", "Public:Error Manager"](reference=w999, error in=w1000, "Public:Module Configuration"=w1003) -> (reference out=w996:refnum<class "Plugin_UI.lvclass">, error out=w994:errorcluster)  [unwired: 1 out]
        n349 = property on="setDefault" class="Bool (strict)"(error in=w994, "DisabledEnum"=T19."Disabled and Grayed Out" ("Disabled")) -> (error out=w992:errorcluster)  [unwired: 1 in, 1 out]
        n350 = Bundle By Name(cluster=w997, "Current Config"=w996, "Initial Config"=w996, "Change Flag"=FALSE ("ChangeFlag")) -> (w995:T11)
      }
      frame "Send Save Response" {
        n351 = call "Send Content Saved Response.vi"("error in (no error)"=w1017, "Configuration UI Event Interface in"=w1020) -> ("error out"=w1019:errorcluster)  [unwired: 8 in, 1 out]
      }
      frame "CheckForUnsavedChanges" {
        # "Check for the changes between initial and current configuration"
        n352 = Unbundle By Name(w1034) -> ("Change Flag"=w1033:bool, "Current Config"=w1035:refnum<class "Plugin_UI.lvclass">, "Initial Config"=w1022:refnum<class "Plugin_UI.lvclass">)
        n353 = Not(x=w1033) -> (.not. x?=w1027:bool)
        n354 = call "Check Unsaved Changes.vi"("error in (no error)"=w1024, "Initial Config"=w1022, "Current Config"=w1035) -> ("error out"=w1023:errorcluster, "No Changes?"=w1026:bool)  [unwired: 7 in]
        n355 = Select(t=T19."Disabled and Grayed Out" ("Disabled"), s=w1026, f=T19."Enabled" ("Disabled")) -> (s? t:f=w1028:T19)
        n356 = And(x=w1027, y=w1026) -> (x .and. y?=w1025:bool)
        n357 = property on="setDefault" class="Bool (strict)"(error in=w1023, "DisabledEnum"=w1028) -> (error out=w1030:errorcluster)  [unwired: 1 in, 1 out]
        n358 = case "No changes" shown="True" w1025 {
          tunnel: w1036 -> [w1039 w1042]
          tunnel: w1030 -> [w1038 w1041]
          tunnel: [w1037 w1040] -> w1029
          frame False {
            # "Send Content changed notification to Test Configurator"
            n359 = call "Send Content Changed.vi"("error in (no error)"=w1038, "Configuration UI Event Interface in"=w1039) -> ("error out"=w1037:errorcluster)  [unwired: 8 in, 1 out]
          }
          frame True {
            # "Send Content unchanged notification to Test Configurator"
            n360 = call "Send Content Unchanged.vi"("error in (no error)"=w1041, "Configuration UI Event Interface in"=w1042) -> ("error out"=w1040:errorcluster)  [unwired: 8 in, 1 out]
          }
        }
      }
      frame "Stop" {
        # "Stop the Plugin"
        n361 = call "Queue Driver.vi"("Queue In"=w1046, "error in (no error)"=w1044, "Operation"=Operation."Release") -> ("error out"=w1047:errorcluster)  [unwired: 9 in, 3 out]
      }
    }
    n362 = Unbundle By Name(w290) -> ("Current Config"=w289:refnum<class "Plugin_UI.lvclass">, "Plugin Name"=w286:string)
    n363 = call <vilib>:"Clear Errors.vi"("error in (no error)"=w284) -> ("error out"=w288:errorcluster)  [unwired: 5 in, 1 out]
    n364 = Format Into String(format string="%s --> %s", error in=w288, w286, w283) -> (resulting string=w285:string)  [unwired: 1 in, 1 out]
    n365 = call-dynamic "Send Error.vi"("Error Level (Warning)"=Error_Levels."Error", "error in"=w284, "Process State"=w285, "Configuration Interface in"=w289) -> ("error out"=w291:errorcluster)  [unwired: 6 in, 1 out]
  }
  n366 = Unbundle By Name(w23) -> ("Current Config"=→"Process out":refnum<class "Plugin_UI.lvclass">)
  n367 = Merge Errors(w16, w17) -> (→"error out":errorcluster)
